vi "UI - BASLER - SINGLE MOTOR high accuracy.vi"() -> ()   [LabVIEW 2015]
uses:
  <vilib>/Utility/miscctls.llb/LVBoundsTypeDef.ctl
  Globals.vi
panel:
  in  "Correlate":bool
  in  "show":bool
  out "merged":picture
  out "fileNameFIBSEM":path
  out "fileNameMergedOPT":path
  in  "Colour 2":u16(ring)=1 items=["561 nm", "488 nm", "404 nm", ""]
  in  "Colour 1":u16(ring) items=["561 nm", "488 nm", "404 nm", ""]
  in  "Two lambda":bool
  in  "abort":bool
  in  "Two lambda old2":bool
  in  "ON/OFF":bool
  in  "Power %":dbl(slide) min=0.0 max=100.0 step=0.1 scale=0.0..100.0 scale format="%1_1f"
  in  "Colour":u16(ring) items=["561 nm", "488 nm", "404 nm", ""]
  in  "moveLAMELLA":bool
  in  "moveFIB":bool
  in  "moveOPT":bool
  in  "Save LAMELLA position":bool
  in  "Save FIB position":bool
  in  "Save OPT position":bool
  in  "Quit TCP":bool
  in  "Grab Image":bool
  out "done":string
  out "data out":string
  out "length":i32
  in  "Grab FIB-SEM":bool
  in  "error Obis":errorcluster
  out "Ready":bool
  in  "moveToOPT":bool
  in  "moveToFIB":bool
  in  "DY mm":dbl=-0.186 format="%.3f"
  in  "DX mm":dbl=49.919 format="%.3f"
  in  "yo":i32=1920
  in  "xo":i32=1200
  in  "yc":i32=2048
  in  "xc":i32=3072
  out "Intensity FIB-SEM":i32[][](graph) caption="Intensity Graph"
  in  "Path to Autoscript":path=path "C:/Program Files/Python35/envs/AutoScript/python.exe"
  in  "FIB/SEM":bool
  in  "Dwell time us":dbl=0.5 format="%#_6f"
  in  "Grab FIB-SEM OLD":bool
  out "wav 1":string
  out "Power":dbl
  in  "Power L1 %":i32(slide) scale=0.0..100.0
  out "LASmouseDOWN":bool
  out "Power1max":dbl
  out "Power1min":dbl
  out "PowerNom1":dbl
  out "lambda":dbl
  out "Obis out":refnum<visa-resource-name>
  in  "baud rate Obis":u32=9600
  out "Message Obis":string
  in  "ON/OFF 3":bool
  out "Obis":bool
  out "L1":bool
  in  "Laser":refnum<visa-resource-name>="COM11"
  out "commando":string
  out "fileName":path
  in  "File Prefix":string="embryo_561nm_"
  out "iii":i32
  in  "StepZ":dbl=1.0 format="%#.3g"
  in  "Nz":i32=50
  in  "startZ":i32=-8000 format="%.3f"
  in  "DIR Series":string="embryo_"
  in  "Scan":bool
  out "Intensity OPT":i32[][](graph) caption="Intensity Graph"
  out "pythonOut":string
  in  "Two lambda grab OLD":bool
  in  "Grab Image OLD":bool
  in  "Path to Python.exe":path=path "C:/Program Files/WinPython-64bit-3.5.4.0Qt5/python-3.5.4.amd64/python.exe"
  in  "Exposure ms":i32=500
  out "Right":bool
  out "Left":bool
  out "Path series":path
  out "date/time string":string="15:37"
  out "systemIndexOut":u32
  out "Path":path=path "C:/Users/Admin/MICROSCOPE/BASLER"
  in  "dz um":dbl=10.0 format="%.3f"
  out "status Z":T1(ring)
  in  "z um":dbl format="%.3f"
  in  "HOME":bool
  in  "STOP":bool
  out "moving":bool
  out "error stage":errorcluster
  out "Z Known?":bool
  in  "System Locator":string="usb:id:199871837"
  # "must be 3.5 for pypylon and basler"
  # "must be 3.5 for pypylon and basler"
  # "×"
  # "×"
  # "from FIB to OPT"
  # "from OPT to FIB"
  # "SEM"
  # "FIB"
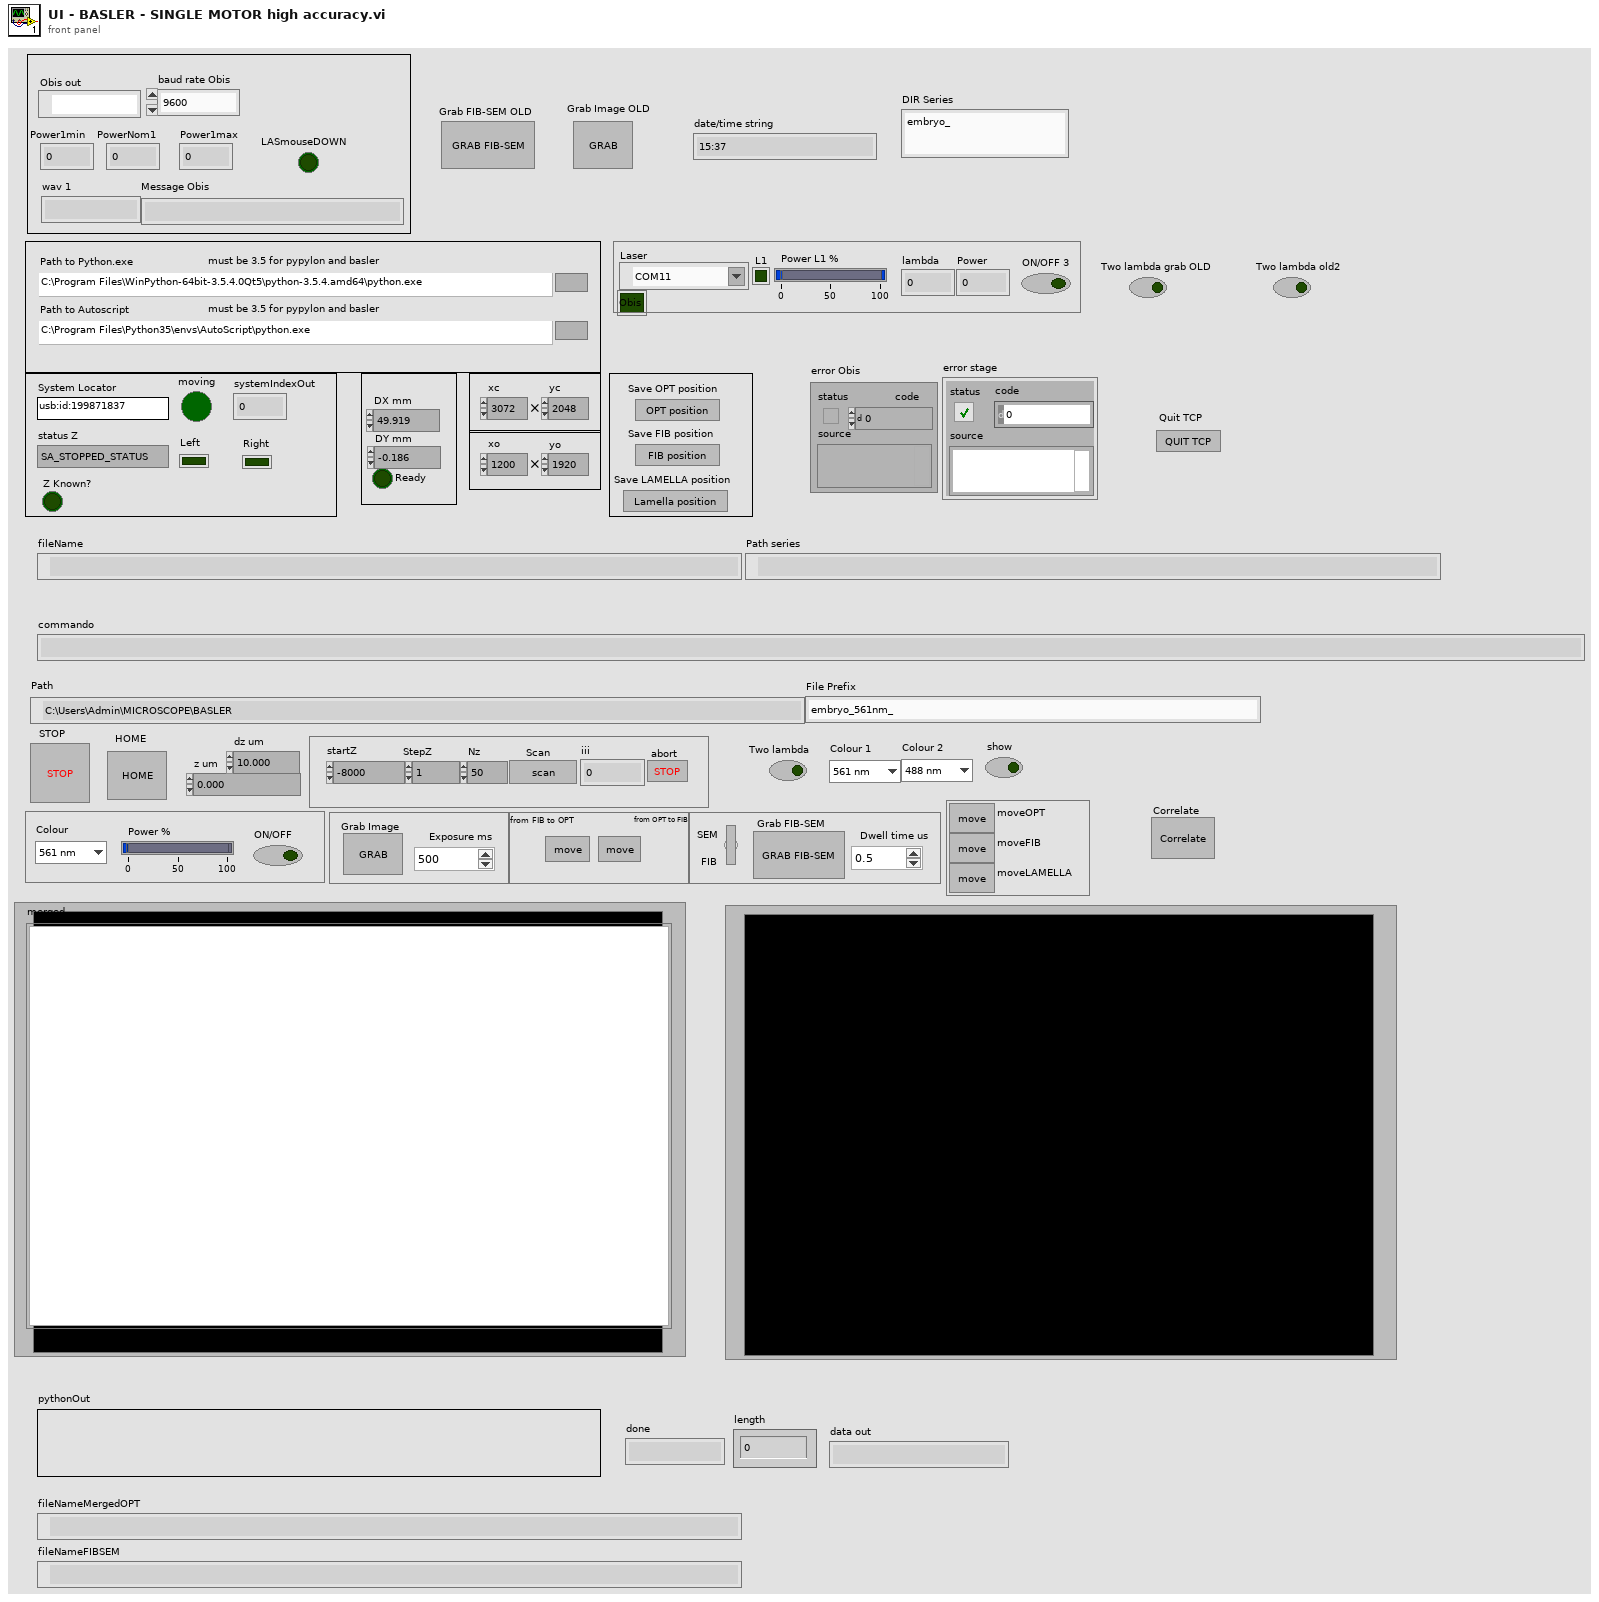
[diagram p1: front panel]
types:
  T1 = enum32{"SA_STOPPED_STATUS", "SA_STEPPING_STATUS", "SA_SCANNING_STATUS", "SA_HOLDING_STATUS", "SA_TARGET_STATUS", "SA_MOVE_DELAY_STATUS", "SA_CALIBRATING_STATUS", "SA_FINDING_REF_STATUS", "SA_OPENING_STATUS"}
  T2 = typedef "LVBoundsTypeDef.ctl" = cluster{"Width":u32, "Height":u32}
  T3 = enum32{"SA_FORWARD_DIRECTION", "SA_BACKWARD_DIRECTION", "SA_FORWARD_BACKWARD_DIRECTION", "SA_BACKWARD_FORWARD_DIRECTION"}
  T4 = typedef "eventvkey.ctl" = enum16{"ASCII", "Enter", "Return", "Shift", "Ctrl", "Alt", "Cmd", "Opt", "Caps", "NumLock", "Clear", "Break", "Up", "Down", "Left", "Right", "Insert", "Delete", "Home", "End", "PageUp", "PageDown", "Escape", "Help", "Pause", "ScrollLock", "F1", "F2", "F3", "F4", "F5", "F6", "F7", "F8", "F9", "F10", "F11", "F12", "F13", "F14", "F15", "F16", "F17", "F18", "F19", "F20", "F21", "F22", "F23", "F24", "Play", "VolumeUp", "VolumeDown", "Mute", "Two Byte Char"}
  T5 = typedef "imagedata.ctl" = cluster{"image type":i32, "image depth":i32, "image":u8[], "mask":u8[], "colors":u32[], "Rectangle":cluster{"left":i16, "top":i16, "right":i16, "bottom":i16}}
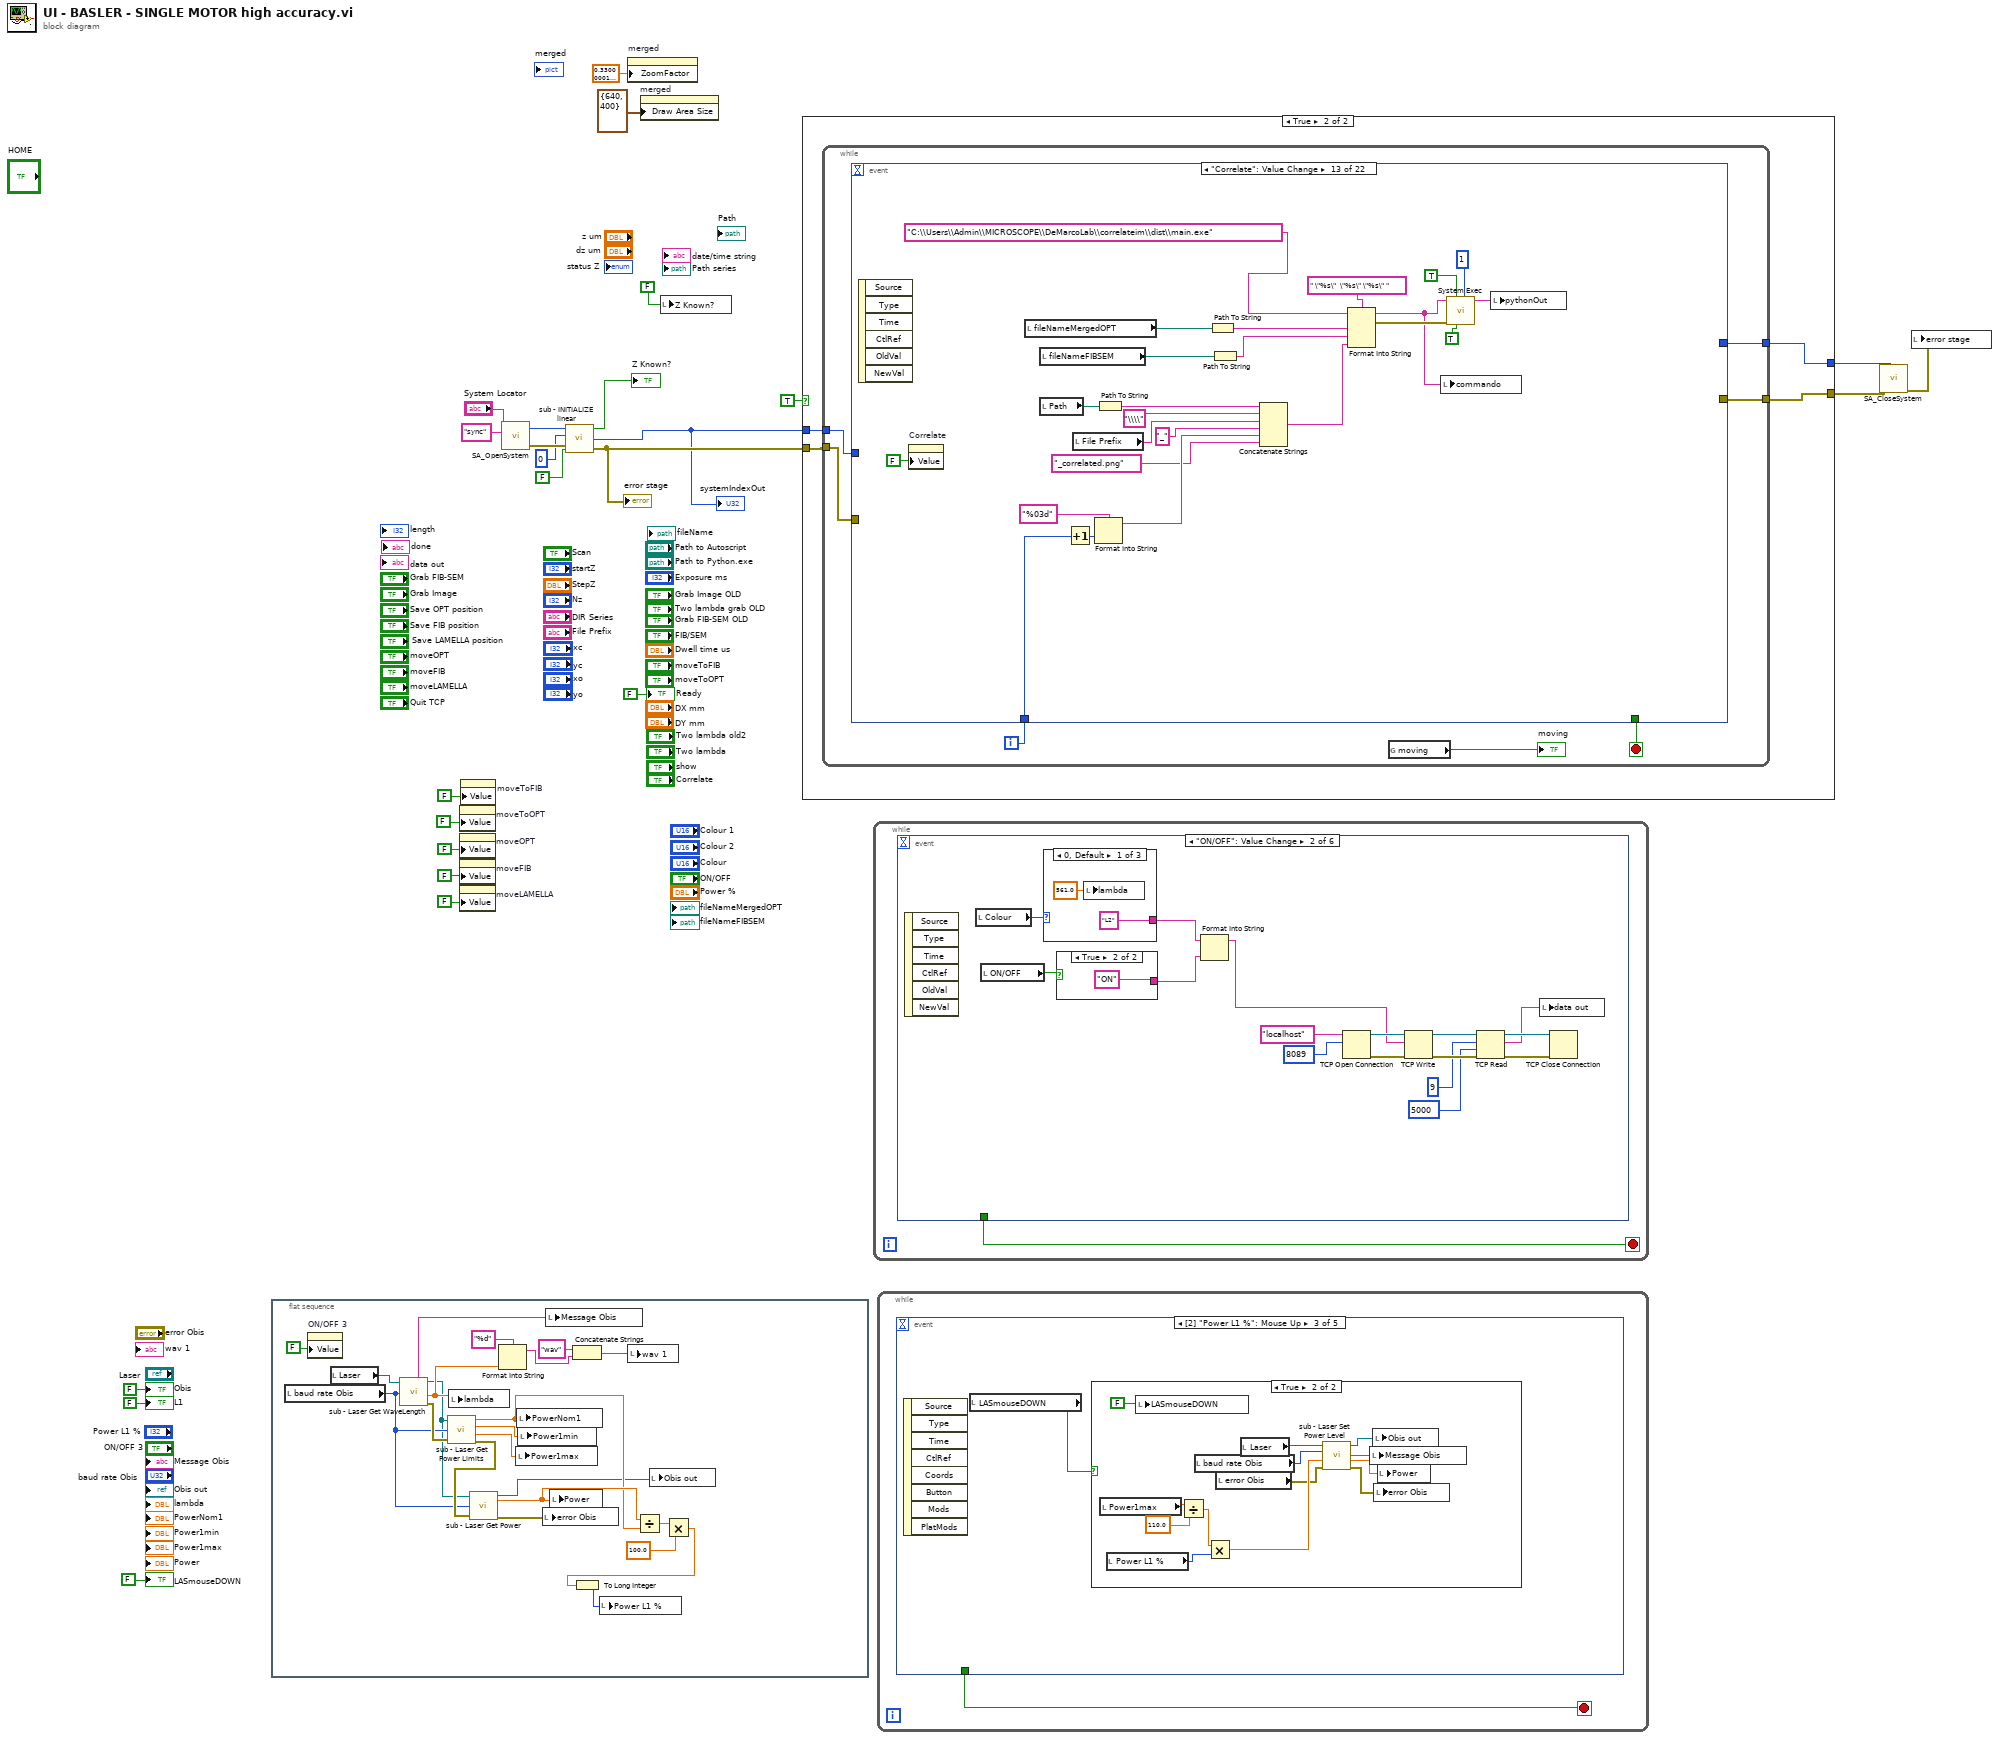
[diagram p0: block diagram]
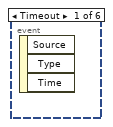
[diagram p2: hidden frame]
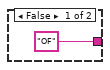
[diagram p3: hidden frame]
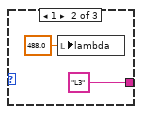
[diagram p4: hidden frame]
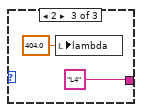
[diagram p5: hidden frame]
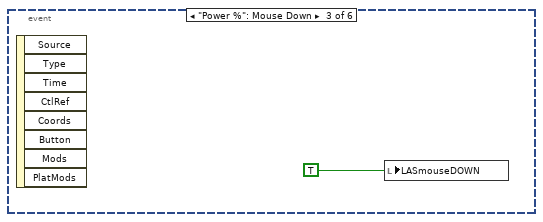
[diagram p6: hidden frame]
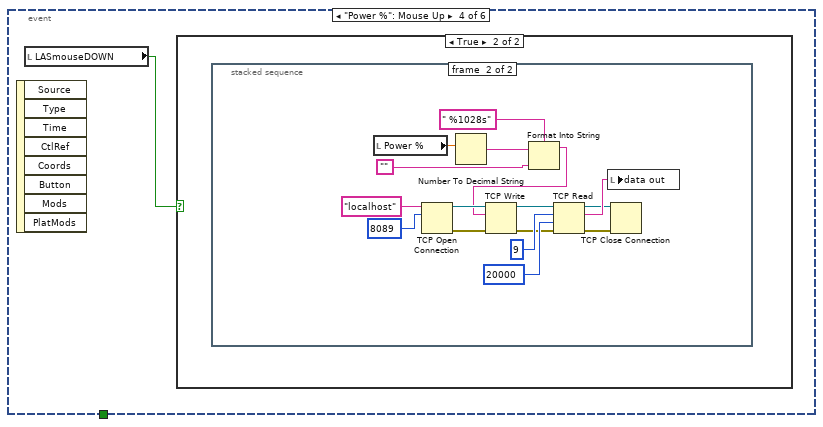
[diagram p7: hidden frame]
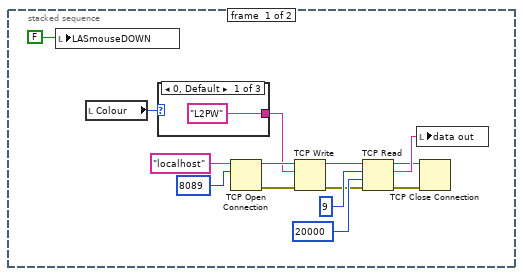
[diagram p9: hidden frame]
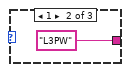
[diagram p10: hidden frame]
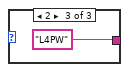
[diagram p11: hidden frame]
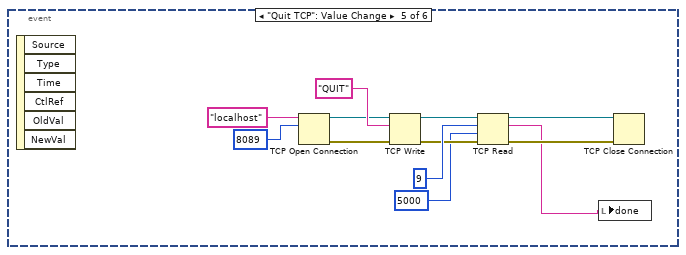
[diagram p12: hidden frame]
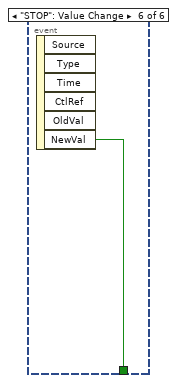
[diagram p13: hidden frame]
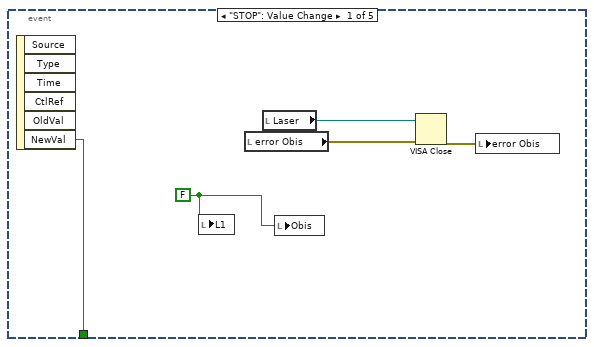
[diagram p14: hidden frame]
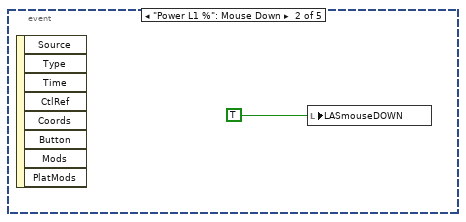
[diagram p15: hidden frame]
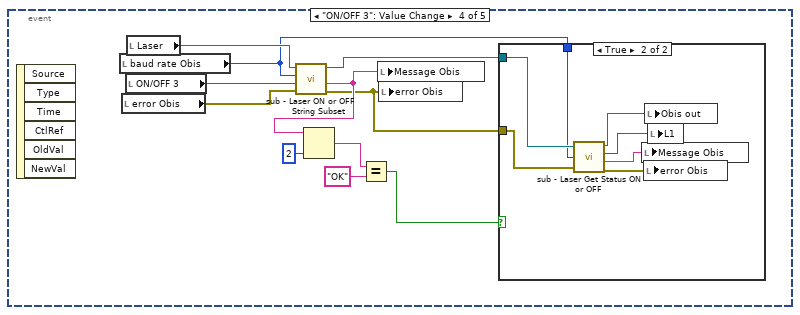
[diagram p17: hidden frame]
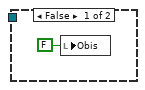
[diagram p18: hidden frame]
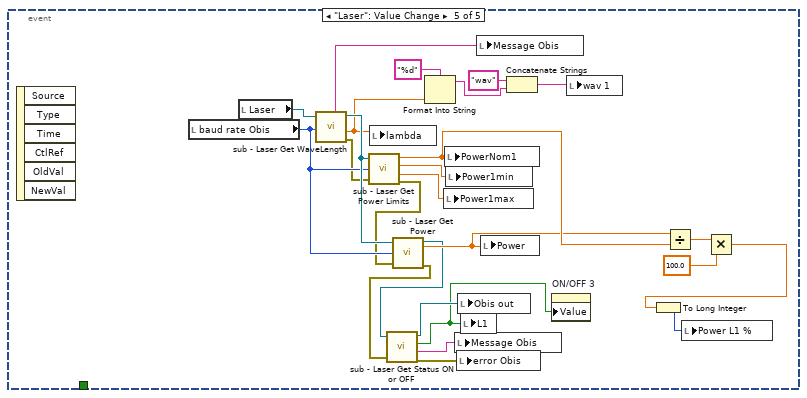
[diagram p19: hidden frame]
diagram:
  n1 = flat-sequence {
    frame #0 {
      n2 = local read "baud rate Obis"() -> (w39:u32)
      n3 = property on="ON/OFF 3" class="Bool (strict)"("Value"=FALSE ("L1 ON/OFF")) -> ()  [unwired: 2 in, 2 out]
      n4 = local read "Laser"() -> (w47:refnum<visa-resource-name>)
      n5 = call "sub - Laser Get WaveLength.vi"("VISA resource name"=w47, "baud rate (9600)"=w39) -> ("reference out"=w28:refnum<visa-resource-name>, "wavelength"=w31:dbl, "error out"=w44:errorcluster, "message"=w45:string)  [unwired: 1 in, 1 out]
      n6 = call "sub - Laser Get Power Limits.vi"("VISA resource name"=w28, "baud rate (9600)"=w39, "error in (no error)"=w44) -> ("powerNominal"=w37:dbl, "powerMin"=w43:dbl, "powerMax"=w42:dbl, "error out"=w41:errorcluster)  [unwired: 1 out]
      n7 = local write "lambda"(w31) -> ()
      n8 = call "sub - Laser Get Power.vi"("VISA resource name"=w28, "baud rate (9600)"=w39, "error in (no error)"=w41) -> ("reference out"=w26:refnum<visa-resource-name>, "Power"=w38:dbl, "error out"=w40:errorcluster)  [unwired: 2 out]
      n9 = Format Into String(format string="%d", w31) -> (resulting string=w27:string)  [unwired: 2 in, 1 out]
      n10 = local write "Power1max"(w42) -> ()
      n11 = local write "PowerNom1"(w37) -> ()
      n12 = local write "Power1min"(w43) -> ()
      n13 = local write "error Obis"(w40) -> ()
      n14 = local write "Message Obis"(w45) -> ()
      n15 = local write "Power"(w38) -> ()
      n16 = Concatenate Strings("wav" ("string"), w27) -> (w29:string)
      n17 = local write "wav 1"(w29) -> ()
      n18 = Divide(x=w38, y=w37) -> (x/y=w36:dbl)
      n19 = local write "Obis out"(w26) -> ()
      n20 = Multiply(x=w36, y=100.0) -> (x*y=w33:dbl)
      n21 = To Long Integer(number=w33) -> (32bit integer=w34:i32)
      n22 = local write "Power L1 %"(w34) -> ()
    }
  }
  n23 = property on="moveToOPT" class="Bool (strict)"("Value"=FALSE ("moveToOPT")) -> ()  [unwired: 2 in, 2 out]
  n24 = property on="moveOPT" class="Bool (strict)"("Value"=FALSE ("moveOPT")) -> ()  [unwired: 2 in, 2 out]
  n25 = property on="moveFIB" class="Bool (strict)"("Value"=FALSE ("moveFIB")) -> ()  [unwired: 2 in, 2 out]
  n26 = property on="moveLAMELLA" class="Bool (strict)"("Value"=FALSE ("moveLAMELLA")) -> ()  [unwired: 2 in, 2 out]
  n27 = property on="moveToFIB" class="Bool (strict)"("Value"=FALSE ("moveToFIB")) -> ()  [unwired: 2 in, 2 out]
  n28 = call <vilib>:"SA_OpenSystem.vi"("options"="sync", "systemLocator"="System Locator") -> ("error out"=w19:errorcluster, "systemIndexOut"=w20:u32)  [unwired: 8 in]
  n29 = call "sub - INITIALIZE linear.vi"("Zero?"=FALSE, "error in (no error)"=w19, "channelIndex"=u32 0, "systemIndex"=w20) -> ("error out"=w15:errorcluster, "systemIndexOut"=w14:u32, "Known?"=→"Z Known?":bool)
  "error stage" <- w15
  "systemIndexOut" <- w14
  n30 = property on="merged" class="Pict"("ZoomFactor"=sgl 0.33 ("Zoom Factor")) -> ()  [unwired: 2 in, 2 out]
  n31 = property on="merged" class="Pict"("Draw Area Size"=T2 {"Width"=640, "Height"=400}) -> ()  [unwired: 2 in, 2 out]
  n32 = local write "Z Known?"(FALSE ("X Known?")) -> ()
  n33 = case shown="True" TRUE {
    tunnel: w14 -> [w49 w53]
    tunnel: [w49 w51] -> w24
    tunnel: w15 -> [w48 w52]
    tunnel: [w48 w50] -> w23
    frame False {
    }
    frame True {
      n34 = while {
        tunnel: w53 -> [w59]
        tunnel: w52 -> [w56]
        tunnel: [w58] -> w51
        tunnel: [w57] -> w50
        i -> [w54]
        stop <- w60 stop-if-true
        n35 = event shown="[12] \"Correlate\": Value Change" {
          selector: _ -> [_ _ _ _ _ _ _ _ _ _ _ _ _ _ _ _ _ _ _ _ _ _]
          dyn-events: _ -> [_ _ _ _ _ _ _ _ _ _ _ _ _ _ _ _ _ _ _ _ _ _]
          timeout: _ -> [_ _ _ _ _ _ _ _ _ _ _ _ _ _ _ _ _ _ _ _ _ _]
          tunnel: [_ _ TRUE _ _ _ _ _ _ _ _ _ _ _ _ _ _ _ _ _ _ FALSE] -> w60
          tunnel: w59 -> [w62 w95 w117 _ _ _ _ _ _ _ _ _ _ _ _ _ _ _ _ _ _ w1778]
          tunnel: w56 -> [w61 w98 w118 _ _ _ _ _ _ _ _ _ _ _ _ _ _ _ _ _ _ w1779]
          tunnel: [_ _ w115 _ _ _ _ _ _ _ _ _ _ _ _ _ _ _ _ _ _ w1778] -> w58
          tunnel: [_ _ w113 _ _ _ _ _ _ _ _ _ _ _ _ _ _ _ _ _ _ _] -> w57
          tunnel: w54 -> [_ _ _ _ _ _ w415 w577 _ w1112 w1440 _ w1577 _ _ _ _ _ _ _ _ _]
          event Key Down {
            n36 = event-data() -> ("VKey"=w63:T4)  [unwired: 1 in, 9 out]
            n37 = case shown="\"Left\"" w63 {
              tunnel: w62 -> [w65 w68 w83]
              tunnel: w61 -> [w64 w66 w81]
              tunnel: [w65 w75 w89] -> _
              tunnel: [w64 w74 w88] -> _
              frame "ASCII", Default {
              }
              frame "Right" {
                n38 = local read "dz um"() -> (w73:dbl)
                n39 = Multiply(x=w73, y=-1) -> (x*y=w67:dbl)
                n40 = call "sub - GoTo Position RELATIVE - HIGH ACCURACY.vi"("error in"=w66, "dx um"=w67, "channelIndex"=u32 0, "systemIndex"=w68) -> ("error out"=w72:errorcluster, "position out um"=w69:dbl, "status"=w71:T1)  [unwired: 2 out]
                n41 = local write "status Z"(w71) -> ()
                n42 = property on="z um" class="DigNum (strict)"("Value"=w69) -> ()  [unwired: 2 in, 2 out]
                n43 = global write "Globals.vi" "X"(w69) -> ()
                n44 = flat-sequence {
                  tunnel: w68 -> [w80]
                  tunnel: [w80] -> w75
                  tunnel: w72 -> [w79]
                  tunnel: [w79] -> w74
                  frame #0 {
                    n45 = local write "Left"(FALSE) -> ()
                  }
                }
                "Left" <- TRUE ("Boolean 2")
              }
              frame "Left" {
                n46 = local read "dz um"() -> (w82:dbl)
                n47 = call "sub - GoTo Position RELATIVE - HIGH ACCURACY.vi"("error in"=w81, "dx um"=w82, "channelIndex"=u32 0, "systemIndex"=w83) -> ("error out"=w86:errorcluster, "position out um"=w84:dbl, "status"=w87:T1)  [unwired: 2 out]
                n48 = local write "status Z"(w87) -> ()
                n49 = global write "Globals.vi" "X"(w84) -> ()
                n50 = property on="z um" class="DigNum (strict)"("Value"=w84) -> ()  [unwired: 2 in, 2 out]
                n51 = flat-sequence {
                  tunnel: w83 -> [w92]
                  tunnel: [w92] -> w89
                  tunnel: w86 -> [w91]
                  tunnel: [w91] -> w88
                  frame #0 {
                    n52 = local write "Right"(FALSE) -> ()
                  }
                }
                "Right" <- TRUE ("Boolean 2")
              }
            }
          }
          event "z um": Value Change {
            n53 = event-data() -> ()  [unwired: 1 in, 6 out]
            n54 = local read "z um"() -> (w97:dbl)
            n55 = call "sub - GoTo Position Absolute ABSOLUTE - HIGH ACCURACY.vi"("error in"=w98, "Position End um"=w97, "channelIndex"=u32 0, "systemIndex"=w95) -> ("error out"=w99:errorcluster, "position out um"=w94:dbl, "status"=w100:T1)  [unwired: 2 out]
            n56 = local write "error stage"(w99) -> ()
            n57 = local write "status Z"(w100) -> ()
            n58 = property on="z um" class="DigNum (strict)"("Value"=w94) -> ()  [unwired: 2 in, 2 out]
          }
          event "STOP": Value Change {
            n59 = event-data() -> ()  [unwired: 1 in, 6 out]
            n60 = flat-sequence {
              tunnel: w118 -> [w125]
              tunnel: w117 -> [w124]
              tunnel: [w122] -> w116
              tunnel: [w121] -> w114
              tunnel: [w140] -> w115
              tunnel: w116 -> [w140]
              tunnel: [w139] -> w113
              tunnel: w114 -> [w139]
              frame #0 {
                w123 = u32 0 ("channelIndex")
                n61 = call <vilib>:"SA_FindReferenceMark_S.vi"("channelIndex"=w123, "systemIndex"=u32 777, "error in (no error)"=w125, "autoZero"=enum32{"SA_NO_AUTO_ZERO", "SA_AUTO_ZERO"}."SA_AUTO_ZERO", "holdTime"=u32 0, "direction"=T3."SA_FORWARD_DIRECTION") -> ("error out"=w129:errorcluster)  [unwired: 5 in]
                n62 = while {
                  tunnel: w124 -> [w135]
                  tunnel: w123 -> [w137]
                  shift-right: [w136] -> w121
                  shift-left: w129 -> [w138]
                  tunnel: [w135] -> w122
                  stop <- w131 stop-if-true
                  n63 = call <vilib>:"SA_GetStatus_S.vi"("channelIndex"=w137, "systemIndex"=u32 777, "error in (no error)"=w138) -> ("error out"=w136:errorcluster, "status"=w134:T1)  [unwired: 7 in]
                  n64 = Equal?(x=T1."SA_STOPPED_STATUS" ("y"), y=w134) -> (x = y?=w131:bool)
                  n65 = Wait (ms)(milliseconds to wait=u32 100) -> ()  [unwired: 1 out]
                }
              }
              frame #1 {
                n66 = global write "Globals.vi" "Stop"("STOP") -> ()
              }
            }
            n67 = TCP Open Connection(address="localhost", remote port or service name=u16 8089) -> (connection ID=w105:refnum<k5>, error out=w104:errorcluster)  [unwired: 3 in]
            n68 = TCP Write(connection ID=w105, data in="QUIT", error in (no error)=w104) -> (connection ID out=w110:refnum<k5>, error out=w109:errorcluster)  [unwired: 1 in, 1 out]
            n69 = TCP Read(connection ID=w110, bytes to read=9, error in (no error)=w109, 9:5000 ("timeout ms (25000)")) -> (connection ID out=w103:refnum<k5>, data out=w101:string, error out=w102:errorcluster)  [unwired: 1 in]
            n70 = local write "done"(w101) -> ()
            n71 = TCP Close Connection(connection ID=w103, error in (no error)=w102) -> ()  [unwired: 1 in, 2 out]
          }
          event "Grab Image OLD": Value Change {
            # "3"
            n72 = event-data() -> ()  [unwired: 1 in, 6 out]
            n73 = local read "Path to Autoscript"() -> (w157:path)
            n74 = local read "Exposure ms"() -> (w155:i32)
            n75 = Multiply(x=w155, y=1000.0) -> (x*y=w154:dbl)
            n76 = Path To String(path=w157) -> (string=w161:string)
            n77 = To Long Integer(number=w154) -> (32bit integer=w153:i32)
            n78 = Format Into String(format string=" \"%s\" %d", initial string=w161, "C:\\Users\\Admin\\MICROSCOPE\\PyPylon_3.5\\camera.py" ("Path to Function"), w153) -> (resulting string=w142:string, error out=w160:errorcluster)  [unwired: 1 in]
            n79 = flat-sequence {
              tunnel: w152 -> [w165]
              tunnel: [w167] -> w146
              frame #0 {
                n80 = Wait (ms)(milliseconds to wait=u32 10) -> ()  [unwired: 1 out]
                "pythonOut" <- w165
              }
              frame #1 {
                n81 = property on="Grab Image OLD" class="Bool (strict)"("Value"=FALSE ("Grab Image")) -> ()  [unwired: 2 in, 2 out]
                n82 = Read from Text File(file (use dialog)=path "C:/Users/Admin/MICROSCOPE/BASLER/dataout.txt" ("file path (dialog if empty)")) -> (text=w167:string)  [unwired: 3 in, 3 out]
              }
            }
            n83 = local write "commando"(w142) -> ()
            n84 = call <vilib>:"System Exec.vi"("run minimized? (F)"=TRUE, "wait until completion? (T)"=TRUE, "error in (no error)"=w160, "command line"=w142) -> ("standard output"=w152:string)  [unwired: 4 in, 3 out]
            n85 = Spreadsheet String To Array(delimiter (Tab)=" ", format string="", spreadsheet string=w146) -> (array=w150:dbl[][])  [unwired: 1 in]
            n86 = local read "yo"() -> (w144:i32)
            n87 = local read "xo"() -> (w143:i32)
            n88 = To Long Integer(number=w150) -> (32bit integer=w149:i32[][])
            n89 = Reshape Array(w149, w144, w143) -> (w151:i32[][])
            n90 = To Long Integer(number=w151) -> (32bit integer=→"Intensity OPT":i32[][])
          }
          event "Scan": Value Change {
            n91 = event-data() -> ()  [unwired: 1 in, 6 out]
            n92 = property on="Scan" class="Bool (strict)"("Value"=FALSE ("Scan")) -> ()  [unwired: 2 in, 2 out]
            n93 = stacked-sequence {
              frame #0 {
                n94 = local read "lambda"() -> (w173:dbl)
                n95 = local read "File Prefix"() -> (w175:string)
                n96 = local read "Path"() -> (w186:path)
                n97 = Number To Decimal String(number=w173) -> (decimal integer string=w172:string)  [unwired: 1 in]
                n98 = Path To String(path=w186) -> (string=w189:string)
                n99 = local read "systemIndexOut"() -> (w178:u32)
                n100 = Format Date/Time String(time format string (%c)="%Y_%m_%d_%H_%M_%S") -> (date/time string=w170:string)  [unwired: 2 in]
                n101 = local read "error stage"() -> (w177:errorcluster)
                n102 = Concatenate Strings(w189, "\\\\" ("format string"), w175, "_SERIES_" ("format string"), w172, "nm__" ("format string"), w170) -> (w188:string)
                n103 = local write "date/time string"(w170) -> ()
                n104 = String To Path(string=w188) -> (path=w187:path)
                n105 = call <vilib>:"Check if File or Folder Exists.vi"("path"=w187) -> ("file or folder exists?"=w185:bool, "dup path"=w184:path)  [unwired: 8 in, 1 out]
                n106 = case shown="False" w185 {
                  tunnel: w184 -> [w192 w194]
                  tunnel: [w193 w194] -> w191
                  frame False {
                    n107 = Create Folder(path (use dialog)=w192) -> (created path=w193:path)  [unwired: 2 in, 2 out]
                  }
                  frame True {
                  }
                }
                n108 = call <vilib>:"SA_GetPosition_S.vi"("channelIndex"=u32 0, "systemIndex"=w178, "error in (no error)"=w177) -> ("error out"=w176:errorcluster, "position"=w181:i32)  [unwired: 7 in]
                n109 = Divide(x=w181, y=1000) -> (x/y=w182:dbl)
                n110 = local write "error stage"(w176) -> ()
                n111 = local write "startZ"(w182) -> ()
                n112 = local write "Path series"(w191) -> ()
              }
              frame #1 {
                n113 = local read "Nz"() -> (w195:i32)
                n114 = for {
                  N: w195 -> [_]
                  i -> [w197]
                  stop <- "abort" stop-if-true
                  n115 = stacked-sequence {
                    frame #0 {
                      # "Move to the position"
                      n116 = local read "StepZ"() -> (w206:dbl)
                      n117 = local read "systemIndexOut"() -> (w200:u32)
                      n118 = local read "error stage"() -> (w203:errorcluster)
                      n119 = local read "iii"() -> (w205:i32)
                      n120 = local read "startZ"() -> (w204:i32)
                      n121 = Multiply(x=w205, y=w206) -> (x*y=w207:dbl)
                      n122 = Add(x=w204, y=w207) -> (x+y=w199:dbl)
                      n123 = call "sub - GoTo Position Absolute ABSOLUTE - HIGH ACCURACY.vi"("error in"=w203, "Position End um"=w199, "channelIndex"=u32 0, "systemIndex"=w200) -> ("position out um"=w198:dbl, "status"=w201:T1)  [unwired: 3 out]
                      n124 = local write "status Z"(w201) -> ()
                      n125 = global write "Globals.vi" "X"(w198) -> ()
                      n126 = property on="z um" class="DigNum (strict)"("Value"=w198) -> ()  [unwired: 2 in, 2 out]
                    }
                    frame #1 {
                      n127 = local read "Path series"() -> (w220:path)
                      n128 = property on="z um" class="DigNum (strict)"() -> ("Value"=w215:dbl)  [unwired: 2 in, 2 out]
                      n129 = local read "iii"() -> (w218:i32)
                      n130 = Increment(x=w218) -> (x+1=w219:i32)
                      n131 = Path To String(path=w220) -> (string=w208:string)
                      n132 = String To Path(string=w208) -> (path=w226:path)
                      n133 = Format Into String(format string="%06f", w215) -> (resulting string=w231:string)  [unwired: 2 in, 1 out]
                      n134 = Format Into String(format string="%03d", w219) -> (resulting string=w217:string)  [unwired: 2 in, 1 out]
                      n135 = call <vilib>:"Check if File or Folder Exists.vi"("path"=w226) -> ("file or folder exists?"=w225:bool, "dup path"=w224:path)  [unwired: 8 in, 1 out]
                      n136 = case shown="False" w225 {
                        tunnel: w224 -> [w232 w234]
                        tunnel: [w233 w234] -> w221
                        frame False {
                          n137 = Create Folder(path (use dialog)=w232) -> (created path=w233:path)  [unwired: 2 in, 2 out]
                        }
                        frame True {
                        }
                      }
                      n138 = Concatenate Strings("_" ("string"), "_" ("string"), w217, "_" ("string"), w231) -> (w211:string)
                      n139 = local read "File Prefix"() -> (w213:string)
                      n140 = Path To String(path=w221) -> (string=w223:string)
                      n141 = Concatenate Strings(w223, "\\\\" ("format string"), w213, "__" ("format string"), w211, ".bmp" ("format string")) -> (w222:string)
                      n142 = String To Path(string=w222) -> (path=w209:path)
                      n143 = local write "fileName"(w209) -> ()
                    }
                    frame #2 {
                      n144 = case shown="True" FALSE {
                        frame False {
                        }
                        frame True {
                          # "U S E   TCP    to send commands"
                          # "OLD WAY TO ACQUIRE IMAGE"
                          n145 = local read "Path series"() -> (w250:path)
                          n146 = local read "Path to Python.exe"() -> (w240:path)
                          n147 = local read "fileName"() -> (w251:path)
                          n148 = local read "Exposure ms"() -> (w238:i32)
                          n149 = Path To String(path=w250) -> (string=w252:string)
                          n150 = Path To String(path=w251) -> (string=w253:string)
                          n151 = Multiply(x=w238, y=1000.0) -> (x*y=w237:dbl)
                          n152 = Path To String(path=w240) -> (string=w245:string)
                          n153 = To Long Integer(number=w237) -> (32bit integer=w236:i32)
                          n154 = Format Into String(format string=" \"%s\" %d \"%s\" \"%s\" \"%s\"", initial string=w245, "C:\\Users\\Admin\\MICROSCOPE\\PyPylon_3.5\\camera.py" ("Path to Function"), w236, "save" ("format string"), w252, w253) -> (resulting string=w242:string, error out=w244:errorcluster)  [unwired: 1 in]
                          "commando" <- w242
                          n155 = call <vilib>:"System Exec.vi"("run minimized? (F)"=TRUE, "wait until completion? (T)"=TRUE, "error in (no error)"=w244, "command line"=w242) -> ("standard output"=w248:string)  [unwired: 4 in, 3 out]
                          n156 = local write "pythonOut"(w248) -> ()
                        }
                      }
                    }
                    frame #3 {
                      n157 = TCP Open Connection(address="localhost", remote port or service name=u16 8089) -> (connection ID=w260:refnum<k5>, error out=w259:errorcluster)  [unwired: 3 in]
                      n158 = TCP Write(connection ID=w260, data in="_OPT" ("format string"), error in (no error)=w259) -> (connection ID out=w265:refnum<k5>, error out=w264:errorcluster)  [unwired: 1 in, 1 out]
                      n159 = TCP Read(connection ID=w265, bytes to read=9, error in (no error)=w264, 9:20000 ("timeout ms (25000)")) -> (connection ID out=w258:refnum<k5>, data out=w255:string, error out=w257:errorcluster)  [unwired: 1 in]
                      n160 = TCP Close Connection(connection ID=w258, error in (no error)=w257) -> ()  [unwired: 1 in, 2 out]
                      n161 = local write "data out"(w255) -> ()
                    }
                    frame #4 {
                      n162 = flat-sequence {
                        frame #0 {
                          n163 = TCP Open Connection(address="localhost", remote port or service name=u16 8089) -> (connection ID=w271:refnum<k5>, error out=w270:errorcluster)  [unwired: 3 in]
                          n164 = TCP Write(connection ID=w271, data in="EXPS", error in (no error)=w270) -> (connection ID out=w276:refnum<k5>, error out=w275:errorcluster)  [unwired: 1 in, 1 out]
                          n165 = TCP Read(connection ID=w276, bytes to read=9, error in (no error)=w275, 9:20000 ("timeout ms (25000)")) -> (connection ID out=w269:refnum<k5>, data out=w266:string, error out=w268:errorcluster)  [unwired: 1 in]
                          n166 = local write "data out"(w266) -> ()
                          n167 = TCP Close Connection(connection ID=w269, error in (no error)=w268) -> ()  [unwired: 1 in, 2 out]
                        }
                        frame #1 {
                          n168 = local read "Exposure ms"() -> (w280:i32)
                          n169 = TCP Open Connection(address="localhost", remote port or service name=u16 8089) -> (connection ID=w287:refnum<k5>, error out=w288:errorcluster)  [unwired: 3 in]
                          n170 = Number To Decimal String(number=w280) -> (decimal integer string=w279:string)  [unwired: 1 in]
                          n171 = Format Into String(format string=" %4s", initial string=w279, "") -> (resulting string=w281:string)  [unwired: 1 in, 1 out]
                          n172 = TCP Write(connection ID=w287, data in=w281, error in (no error)=w288) -> (connection ID out=w282:refnum<k5>, error out=w283:errorcluster)  [unwired: 1 in, 1 out]
                          n173 = TCP Read(connection ID=w282, bytes to read=9, error in (no error)=w283, 9:20000 ("timeout ms (25000)")) -> (connection ID out=w289:refnum<k5>, data out=w292:string, error out=w290:errorcluster)  [unwired: 1 in]
                          n174 = local write "data out"(w292) -> ()
                          n175 = TCP Close Connection(connection ID=w289, error in (no error)=w290) -> ()  [unwired: 1 in, 2 out]
                        }
                      }
                    }
                    frame #5 {
                      n176 = flat-sequence {
                        frame #0 {
                          n177 = TCP Open Connection(address="localhost", remote port or service name=u16 8089) -> (connection ID=w299:refnum<k5>, error out=w298:errorcluster)  [unwired: 3 in]
                          n178 = TCP Write(connection ID=w299, data in="_DIR", error in (no error)=w298) -> (connection ID out=w304:refnum<k5>, error out=w303:errorcluster)  [unwired: 1 in, 1 out]
                          n179 = TCP Read(connection ID=w304, bytes to read=9, error in (no error)=w303, 9:20000 ("timeout ms (25000)")) -> (connection ID out=w297:refnum<k5>, data out=w294:string, error out=w296:errorcluster)  [unwired: 1 in]
                          n180 = local write "data out"(w294) -> ()
                          n181 = TCP Close Connection(connection ID=w297, error in (no error)=w296) -> ()  [unwired: 1 in, 2 out]
                        }
                        frame #1 {
                          n182 = local read "fileName"() -> (w310:path)
                          n183 = Path To String(path=w310) -> (string=w308:string)
                          n184 = TCP Open Connection(address="localhost", remote port or service name=u16 8089) -> (connection ID=w316:refnum<k5>, error out=w317:errorcluster)  [unwired: 3 in]
                          n185 = Format Into String(format string=" %1028s", initial string=w308, "") -> (resulting string=w309:string)  [unwired: 1 in, 1 out]
                          n186 = TCP Write(connection ID=w316, data in=w309, error in (no error)=w317) -> (connection ID out=w311:refnum<k5>, error out=w312:errorcluster)  [unwired: 1 in, 1 out]
                          n187 = TCP Read(connection ID=w311, bytes to read=9, error in (no error)=w312, 9:20000 ("timeout ms (25000)")) -> (connection ID out=w318:refnum<k5>, data out=w321:string, error out=w319:errorcluster)  [unwired: 1 in]
                          n188 = local write "data out"(w321) -> ()
                          n189 = TCP Close Connection(connection ID=w318, error in (no error)=w319) -> ()  [unwired: 1 in, 2 out]
                        }
                      }
                    }
                    frame #6 {
                      n190 = TCP Open Connection(address="localhost", remote port or service name=u16 8089) -> (connection ID=w327:refnum<k5>, error out=w326:errorcluster)  [unwired: 3 in]
                      n191 = TCP Write(connection ID=w327, data in="IMGO", error in (no error)=w326) -> (connection ID out=w332:refnum<k5>, error out=w331:errorcluster)  [unwired: 1 in, 1 out]
                      n192 = TCP Read(connection ID=w332, bytes to read=9, error in (no error)=w331, 9:20000 ("timeout ms (25000)")) -> (connection ID out=w325:refnum<k5>, data out=w322:string, error out=w324:errorcluster)  [unwired: 1 in]
                      n193 = TCP Close Connection(connection ID=w325, error in (no error)=w324) -> ()  [unwired: 1 in, 2 out]
                      n194 = local write "data out"(w322) -> ()
                    }
                    frame #7 {
                      n195 = TCP Open Connection(address="localhost", remote port or service name=u16 8089) -> (connection ID=w340:refnum<k5>, error out=w339:errorcluster)  [unwired: 3 in]
                      n196 = TCP Write(connection ID=w340, data in="GETL", error in (no error)=w339) -> (connection ID out=w345:refnum<k5>, error out=w344:errorcluster)  [unwired: 1 in, 1 out]
                      n197 = TCP Read(connection ID=w345, bytes to read=20, error in (no error)=w344, 9:5000 ("timeout ms (25000)")) -> (connection ID out=w338:refnum<k5>, data out=w335:string, error out=w337:errorcluster)  [unwired: 1 in]
                      n198 = Decimal String To Number(string=w335) -> (number=w334:i32)  [unwired: 2 in, 1 out]
                      n199 = local write "data out"(w335) -> ()
                      n200 = TCP Close Connection(connection ID=w338, error in (no error)=w337) -> ()  [unwired: 1 in, 2 out]
                      n201 = local write "length"(w334) -> ()
                    }
                    frame #8 {
                      n202 = local read "length"() -> (w363:i32)
                      n203 = TCP Open Connection(address="localhost", remote port or service name=u16 8089) -> (connection ID=w361:refnum<k5>, error out=w362:errorcluster)  [unwired: 3 in]
                      n204 = TCP Write(connection ID=w361, data in="DATA", error in (no error)=w362) -> (connection ID out=w356:refnum<k5>, error out=w357:errorcluster)  [unwired: 1 in, 1 out]
                      n205 = TCP Read(connection ID=w356, bytes to read=w363, error in (no error)=w357, 9:5000 ("timeout ms (25000)")) -> (data out=w347:string)  [unwired: 1 in, 2 out]
                      n206 = Spreadsheet String To Array(delimiter (Tab)=" ", format string="", spreadsheet string=w347) -> (array=w353:dbl[][])  [unwired: 1 in]
                      n207 = local read "yo"() -> (w348:i32)
                      n208 = local read "xo"() -> (w349:i32)
                      n209 = To Long Integer(number=w353) -> (32bit integer=w352:i32[][])
                      n210 = Reshape Array(w352, w348, w349) -> (w354:i32[][])
                      n211 = To Long Integer(number=w354) -> (32bit integer=w364:i32[][])
                      n212 = local write "Intensity OPT"(w364) -> ()
                    }
                  }
                  "iii" <- w197
                }
              }
            }
          }
          event "Grab FIB-SEM OLD": Value Change {
            n213 = event-data() -> ()  [unwired: 1 in, 6 out]
            n214 = stacked-sequence {
              frame #0 {
                n215 = local read "FIB/SEM"() -> (w366:bool)
                n216 = case shown="True" w366 {
                  tunnel: ["_FIB_" ("format string") "_SEM_" ("format string")] -> w365
                  frame False {
                  }
                  frame True {
                  }
                }
                n217 = local read "File Prefix"() -> (w368:string)
                n218 = local read "Path"() -> (w372:path)
                n219 = Path To String(path=w372) -> (string=w375:string)
                n220 = Format Date/Time String(time format string (%c)="%Y_%m_%d_%H_%M_%S") -> (date/time string=w367:string)  [unwired: 2 in]
                n221 = Concatenate Strings(w375, "\\\\" ("format string"), w368, w365, w367) -> (w374:string)
                n222 = local write "date/time string"(w367) -> ()
                n223 = String To Path(string=w374) -> (path=w373:path)
                n224 = call <vilib>:"Check if File or Folder Exists.vi"("path"=w373) -> ("file or folder exists?"=w371:bool, "dup path"=w370:path)  [unwired: 8 in, 1 out]
                n225 = case shown="False" w371 {
                  tunnel: w370 -> [w380 w382]
                  tunnel: [w381 w382] -> w377
                  frame False {
                    n226 = Create Folder(path (use dialog)=w380) -> (created path=w381:path)  [unwired: 2 in, 2 out]
                  }
                  frame True {
                  }
                }
                n227 = local write "Path series"(w377) -> ()
              }
              frame #1 {
                n228 = local read "FIB/SEM"() -> (w389:bool)
                n229 = case shown="False" w389 {
                  tunnel: ["C:\\Users\\Admin\\MICROSCOPE\\pfib__GetFIBimage.py" ("Path to Function") "C:\\Users\\Admin\\MICROSCOPE\\pfib__GetSEMimage.py" ("Path to Function")] -> w388
                  frame False {
                  }
                  frame True {
                  }
                }
                n230 = local read "File Prefix"() -> (w387:string)
                n231 = local read "Path series"() -> (w397:path)
                n232 = local read "Path to Autoscript"() -> (w390:path)
                n233 = local read "Dwell time us"() -> (w384:dbl)
                n234 = Path To String(path=w397) -> (string=w398:string)
                n235 = Path To String(path=w390) -> (string=w394:string)
                n236 = Format Into String(format string=" \"%s\" %f \"%s\" \"%s\" \"%s\"", initial string=w394, w388, w384, w387, w398, "plot" ("Path to Function")) -> (resulting string=w385:string, error out=w393:errorcluster)  [unwired: 1 in]
                n237 = local write "commando"(w385) -> ()
                n238 = call <vilib>:"System Exec.vi"("expected output size  (4096)"=u32 1, "run minimized? (F)"=TRUE, "wait until completion? (T)"=TRUE, "error in (no error)"=w393, "command line"=w385) -> ("standard output"=w396:string)  [unwired: 3 in, 3 out]
                n239 = local write "pythonOut"(w396) -> ()
              }
              frame #2 {
                n240 = local read "FIB/SEM"() -> (w412:bool)
                n241 = property on="Grab FIB-SEM OLD" class="Bool (strict)"("Value"=FALSE ("Grab Image")) -> ()  [unwired: 2 in, 2 out]
                n242 = case shown="True" w412 {
                  tunnel: [path "C:/Users/Admin/MICROSCOPE/BASLER/dataoutFIB.txt" ("file path (dialog if empty)") path "C:/Users/Admin/MICROSCOPE/BASLER/dataoutSEM.txt" ("file path (dialog if empty)")] -> w411
                  frame False {
                  }
                  frame True {
                  }
                }
                n243 = local read "xc"() -> (w401:i32)
                n244 = local read "yc"() -> (w402:i32)
                n245 = Read from Text File(file (use dialog)=w411) -> (text=w403:string)  [unwired: 3 in, 3 out]
                n246 = Spreadsheet String To Array(delimiter (Tab)=" ", format string="", spreadsheet string=w403) -> (array=w408:dbl[][])  [unwired: 1 in]
                n247 = To Long Integer(number=w408) -> (32bit integer=w407:i32[][])
                n248 = Reshape Array(w407, w401, w402) -> (w409:i32[][])
                n249 = To Long Integer(number=w409) -> (32bit integer=→"Intensity FIB-SEM":i32[][])
              }
            }
          }
          event "Grab FIB-SEM": Value Change {
            n250 = event-data() -> ()  [unwired: 1 in, 6 out]
            n251 = stacked-sequence {
              tunnel: w415 -> [w419 _ _ _ _ _ _ _ _]
              frame #0 {
                n252 = local read "FIB/SEM"() -> (w424:bool)
                n253 = local read "Path"() -> (w428:path)
                n254 = case shown="True" w424 {
                  tunnel: ["_FIB_" ("format string") "_SEM_" ("format string")] -> w416
                  frame False {
                  }
                  frame True {
                  }
                }
                n255 = local read "File Prefix"() -> (w426:string)
                n256 = Path To String(path=w428) -> (string=w431:string)
                n257 = Increment(x=w419) -> (x+1=w420:i32)
                n258 = Format Into String(format string="%03d", w420) -> (resulting string=w417:string)  [unwired: 2 in, 1 out]
                n259 = Format Date/Time String(time format string (%c)="%Y_%m_%d_%H_%M_%S") -> (date/time string=w425:string)  [unwired: 2 in]
                n260 = local write "date/time string"(w425) -> ()
                n261 = Concatenate Strings(w431, "\\\\" ("format string"), w426, "_" ("format string"), w417, w416) -> (w430:string)
                n262 = String To Path(string=w430) -> (path=w429:path)
                n263 = call <vilib>:"Check if File or Folder Exists.vi"("path"=w429) -> ("dup path"=w422:path)  [unwired: 8 in, 2 out]
                n264 = case shown="True" TRUE {
                  tunnel: w422 -> [w435 w437]
                  tunnel: [w436 w437] -> _
                  frame False {
                    n265 = Create Folder(path (use dialog)=w435) -> (created path=w436:path)  [unwired: 2 in, 2 out]
                  }
                  frame True {
                  }
                }
                n266 = local write "fileName"(w422) -> ()
              }
              frame #1 {
                n267 = local read "FIB/SEM"() -> (w439:bool)
                n268 = case shown="False" w439 {
                  tunnel: ["_FIB" ("format string") "_SEM" ("format string")] -> w438
                  frame False {
                  }
                  frame True {
                  }
                }
                n269 = TCP Open Connection(address="localhost", remote port or service name=u16 8089) -> (connection ID=w445:refnum<k5>, error out=w444:errorcluster)  [unwired: 3 in]
                n270 = TCP Write(connection ID=w445, data in=w438, error in (no error)=w444) -> (connection ID out=w450:refnum<k5>, error out=w449:errorcluster)  [unwired: 1 in, 1 out]
                n271 = TCP Read(connection ID=w450, bytes to read=9, error in (no error)=w449, 9:20000 ("timeout ms (25000)")) -> (connection ID out=w443:refnum<k5>, data out=w440:string, error out=w442:errorcluster)  [unwired: 1 in]
                n272 = TCP Close Connection(connection ID=w443, error in (no error)=w442) -> ()  [unwired: 1 in, 2 out]
                n273 = local write "data out"(w440) -> ()
              }
              frame #2 {
                n274 = flat-sequence {
                  frame #0 {
                    n275 = TCP Open Connection(address="localhost", remote port or service name=u16 8089) -> (connection ID=w458:refnum<k5>, error out=w457:errorcluster)  [unwired: 3 in]
                    n276 = TCP Write(connection ID=w458, data in="DWEL", error in (no error)=w457) -> (connection ID out=w463:refnum<k5>, error out=w462:errorcluster)  [unwired: 1 in, 1 out]
                    n277 = TCP Read(connection ID=w463, bytes to read=9, error in (no error)=w462, 9:20000 ("timeout ms (25000)")) -> (connection ID out=w456:refnum<k5>, data out=w453:string, error out=w455:errorcluster)  [unwired: 1 in]
                    n278 = local write "data out"(w453) -> ()
                    n279 = TCP Close Connection(connection ID=w456, error in (no error)=w455) -> ()  [unwired: 1 in, 2 out]
                  }
                  frame #1 {
                    n280 = local read "Dwell time us"() -> (w477:dbl)
                    n281 = TCP Open Connection(address="localhost", remote port or service name=u16 8089) -> (connection ID=w471:refnum<k5>, error out=w472:errorcluster)  [unwired: 3 in]
                    n282 = Format Into String(format string=" %1.2f", initial string="", w477) -> (resulting string=w465:string)  [unwired: 1 in, 1 out]
                    n283 = TCP Write(connection ID=w471, data in=w465, error in (no error)=w472) -> (connection ID out=w466:refnum<k5>, error out=w467:errorcluster)  [unwired: 1 in, 1 out]
                    n284 = TCP Read(connection ID=w466, bytes to read=9, error in (no error)=w467, 9:20000 ("timeout ms (25000)")) -> (connection ID out=w473:refnum<k5>, data out=w476:string, error out=w474:errorcluster)  [unwired: 1 in]
                    n285 = local write "data out"(w476) -> ()
                    n286 = TCP Close Connection(connection ID=w473, error in (no error)=w474) -> ()  [unwired: 1 in, 2 out]
                  }
                }
              }
              frame #3 {
                n287 = flat-sequence {
                  frame #0 {
                    n288 = TCP Open Connection(address="localhost", remote port or service name=u16 8089) -> (connection ID=w485:refnum<k5>, error out=w484:errorcluster)  [unwired: 3 in]
                    n289 = TCP Write(connection ID=w485, data in="_DIR", error in (no error)=w484) -> (connection ID out=w490:refnum<k5>, error out=w489:errorcluster)  [unwired: 1 in, 1 out]
                    n290 = TCP Read(connection ID=w490, bytes to read=9, error in (no error)=w489, 9:20000 ("timeout ms (25000)")) -> (connection ID out=w483:refnum<k5>, data out=w480:string, error out=w482:errorcluster)  [unwired: 1 in]
                    n291 = local write "data out"(w480) -> ()
                    n292 = TCP Close Connection(connection ID=w483, error in (no error)=w482) -> ()  [unwired: 1 in, 2 out]
                  }
                  frame #1 {
                    n293 = local read "fileName"() -> (w496:path)
                    n294 = Path To String(path=w496) -> (string=w494:string)
                    n295 = TCP Open Connection(address="localhost", remote port or service name=u16 8089) -> (connection ID=w502:refnum<k5>, error out=w503:errorcluster)  [unwired: 3 in]
                    n296 = Format Into String(format string=" %1028s", initial string=w494, "") -> (resulting string=w495:string)  [unwired: 1 in, 1 out]
                    n297 = TCP Write(connection ID=w502, data in=w495, error in (no error)=w503) -> (connection ID out=w497:refnum<k5>, error out=w498:errorcluster)  [unwired: 1 in, 1 out]
                    n298 = TCP Read(connection ID=w497, bytes to read=9, error in (no error)=w498, 9:20000 ("timeout ms (25000)")) -> (connection ID out=w504:refnum<k5>, data out=w507:string, error out=w505:errorcluster)  [unwired: 1 in]
                    n299 = local write "data out"(w507) -> ()
                    n300 = TCP Close Connection(connection ID=w504, error in (no error)=w505) -> ()  [unwired: 1 in, 2 out]
                  }
                }
              }
              frame #4 {
                n301 = TCP Open Connection(address="localhost", remote port or service name=u16 8089) -> (connection ID=w513:refnum<k5>, error out=w512:errorcluster)  [unwired: 3 in]
                n302 = TCP Write(connection ID=w513, data in="IMGS", error in (no error)=w512) -> (connection ID out=w518:refnum<k5>, error out=w517:errorcluster)  [unwired: 1 in, 1 out]
                n303 = TCP Read(connection ID=w518, bytes to read=9, error in (no error)=w517, 9:20000 ("timeout ms (25000)")) -> (connection ID out=w511:refnum<k5>, data out=w508:string, error out=w510:errorcluster)  [unwired: 1 in]
                n304 = TCP Close Connection(connection ID=w511, error in (no error)=w510) -> ()  [unwired: 1 in, 2 out]
                n305 = local write "data out"(w508) -> ()
              }
              frame #5 {
                n306 = TCP Open Connection(address="localhost", remote port or service name=u16 8089) -> (connection ID=w526:refnum<k5>, error out=w525:errorcluster)  [unwired: 3 in]
                n307 = TCP Write(connection ID=w526, data in="GETL", error in (no error)=w525) -> (connection ID out=w531:refnum<k5>, error out=w530:errorcluster)  [unwired: 1 in, 1 out]
                n308 = TCP Read(connection ID=w531, bytes to read=20, error in (no error)=w530, 9:5000 ("timeout ms (25000)")) -> (connection ID out=w524:refnum<k5>, data out=w521:string, error out=w523:errorcluster)  [unwired: 1 in]
                n309 = Decimal String To Number(string=w521) -> (number=w520:i32)  [unwired: 2 in, 1 out]
                n310 = local write "data out"(w521) -> ()
                n311 = local write "length"(w520) -> ()
                n312 = TCP Close Connection(connection ID=w524, error in (no error)=w523) -> ()  [unwired: 1 in, 2 out]
              }
              frame #6 {
                n313 = property on="Grab FIB-SEM OLD" class="Bool (strict)"("Value"=FALSE ("Grab Image")) -> ()  [unwired: 2 in, 2 out]
                n314 = TCP Open Connection(address="localhost", remote port or service name=u16 8089) -> (connection ID=w549:refnum<k5>, error out=w550:errorcluster)  [unwired: 3 in]
                n315 = local read "length"() -> (w551:i32)
                n316 = TCP Write(connection ID=w549, data in="DATA", error in (no error)=w550) -> (connection ID out=w544:refnum<k5>, error out=w545:errorcluster)  [unwired: 1 in, 1 out]
                n317 = TCP Read(connection ID=w544, bytes to read=w551, error in (no error)=w545, 9:5000 ("timeout ms (25000)")) -> (data out=w534:string)  [unwired: 1 in, 2 out]
                n318 = Spreadsheet String To Array(delimiter (Tab)=" ", format string="", spreadsheet string=w534) -> (array=w540:dbl[][])  [unwired: 1 in]
                n319 = local read "xc"() -> (w535:i32)
                n320 = local read "yc"() -> (w536:i32)
                n321 = To Long Integer(number=w540) -> (32bit integer=w539:i32[][])
                n322 = Reshape Array(w539, w535, w536) -> (w541:i32[][])
                n323 = To Long Integer(number=w541) -> (32bit integer=w542:i32[][])
                n324 = local write "Intensity FIB-SEM"(w542) -> ()
              }
              frame #7 {
                # "what is the length of the data - PATH?"
                n325 = property on="Grab FIB-SEM" class="Bool (strict)"("Value"=FALSE ("Grab FIB-SEM TCP")) -> ()  [unwired: 2 in, 2 out]
                n326 = TCP Open Connection(address="localhost", remote port or service name=u16 8089) -> (connection ID=w558:refnum<k5>, error out=w557:errorcluster)  [unwired: 3 in]
                n327 = TCP Write(connection ID=w558, data in="GLPT", error in (no error)=w557) -> (connection ID out=w563:refnum<k5>, error out=w562:errorcluster)  [unwired: 1 in, 1 out]
                n328 = TCP Read(connection ID=w563, bytes to read=20, error in (no error)=w562, 9:5000 ("timeout ms (25000)")) -> (connection ID out=w556:refnum<k5>, data out=w553:string, error out=w555:errorcluster)  [unwired: 1 in]
                n329 = Decimal String To Number(string=w553) -> (number=w552:i32)  [unwired: 2 in, 1 out]
                n330 = local write "data out"(w553) -> ()
                n331 = TCP Close Connection(connection ID=w556, error in (no error)=w555) -> ()  [unwired: 1 in, 2 out]
                n332 = local write "length"(w552) -> ()
              }
              frame #8 {
                # "file path to the merged bmp"
                n333 = TCP Open Connection(address="localhost", remote port or service name=u16 8089) -> (connection ID=w574:refnum<k5>, error out=w575:errorcluster)  [unwired: 3 in]
                n334 = local read "length"() -> (w576:i32)
                n335 = TCP Write(connection ID=w574, data in="DTPH", error in (no error)=w575) -> (connection ID out=w569:refnum<k5>, error out=w570:errorcluster)  [unwired: 1 in, 1 out]
                n336 = TCP Read(connection ID=w569, bytes to read=w576, error in (no error)=w570, 9:5000 ("timeout ms (25000)")) -> (data out=w567:string)  [unwired: 1 in, 2 out]
                n337 = String To Path(string=w567) -> (path=w566:path)
                n338 = local write "pythonOut"(w567) -> ()
                n339 = local write "fileNameFIBSEM"(w566) -> ()
              }
            }
          }
          event "Grab Image": Value Change {
            n340 = event-data() -> ()  [unwired: 1 in, 6 out]
            n341 = stacked-sequence {
              tunnel: w577 -> [w582 _ _ _ _ _ _ _]
              frame #0 {
                w578 = "_" ("format string")
                n342 = local read "lambda"() -> (w586:dbl)
                n343 = local read "Path"() -> (w591:path)
                n344 = local read "File Prefix"() -> (w589:string)
                n345 = Number To Decimal String(number=w586) -> (decimal integer string=w579:string)  [unwired: 1 in]
                n346 = Increment(x=w582) -> (x+1=w583:i32)
                n347 = Path To String(path=w591) -> (string=w594:string)
                n348 = Format Into String(format string="%03d", w583) -> (resulting string=w581:string)  [unwired: 2 in, 1 out]
                n349 = Format Date/Time String(time format string (%c)="%Y_%m_%d_%H_%M_%S") -> (date/time string=w585:string)  [unwired: 2 in]
                n350 = local write "date/time string"(w585) -> ()
                n351 = Concatenate Strings(w594, "\\\\" ("format string"), w589, w578, w581, "_OPT_" ("format string"), w579, w578) -> (w593:string)
                n352 = String To Path(string=w593) -> (path=w592:path)
                n353 = call <vilib>:"Check if File or Folder Exists.vi"("path"=w592) -> ("dup path"=w587:path)  [unwired: 8 in, 2 out]
                n354 = case shown="True" TRUE {
                  tunnel: w587 -> [w596 w598]
                  tunnel: [w597 w598] -> _
                  frame False {
                    n355 = Create Folder(path (use dialog)=w596) -> (created path=w597:path)  [unwired: 2 in, 2 out]
                  }
                  frame True {
                  }
                }
                n356 = local write "fileName"(w587) -> ()
              }
              frame #1 {
                n357 = TCP Open Connection(address="localhost", remote port or service name=u16 8089) -> (connection ID=w605:refnum<k5>, error out=w604:errorcluster)  [unwired: 3 in]
                n358 = TCP Write(connection ID=w605, data in="_OPT" ("format string"), error in (no error)=w604) -> (connection ID out=w610:refnum<k5>, error out=w609:errorcluster)  [unwired: 1 in, 1 out]
                n359 = TCP Read(connection ID=w610, bytes to read=9, error in (no error)=w609, 9:20000 ("timeout ms (25000)")) -> (connection ID out=w603:refnum<k5>, data out=w600:string, error out=w602:errorcluster)  [unwired: 1 in]
                n360 = TCP Close Connection(connection ID=w603, error in (no error)=w602) -> ()  [unwired: 1 in, 2 out]
                n361 = local write "data out"(w600) -> ()
              }
              frame #2 {
                n362 = flat-sequence {
                  frame #0 {
                    n363 = TCP Open Connection(address="localhost", remote port or service name=u16 8089) -> (connection ID=w616:refnum<k5>, error out=w615:errorcluster)  [unwired: 3 in]
                    n364 = TCP Write(connection ID=w616, data in="EXPS", error in (no error)=w615) -> (connection ID out=w621:refnum<k5>, error out=w620:errorcluster)  [unwired: 1 in, 1 out]
                    n365 = TCP Read(connection ID=w621, bytes to read=9, error in (no error)=w620, 9:20000 ("timeout ms (25000)")) -> (connection ID out=w614:refnum<k5>, data out=w611:string, error out=w613:errorcluster)  [unwired: 1 in]
                    n366 = local write "data out"(w611) -> ()
                    n367 = TCP Close Connection(connection ID=w614, error in (no error)=w613) -> ()  [unwired: 1 in, 2 out]
                  }
                  frame #1 {
                    n368 = local read "Exposure ms"() -> (w625:i32)
                    n369 = TCP Open Connection(address="localhost", remote port or service name=u16 8089) -> (connection ID=w632:refnum<k5>, error out=w633:errorcluster)  [unwired: 3 in]
                    n370 = Number To Decimal String(number=w625) -> (decimal integer string=w624:string)  [unwired: 1 in]
                    n371 = Format Into String(format string=" %4s", initial string=w624, "") -> (resulting string=w626:string)  [unwired: 1 in, 1 out]
                    n372 = TCP Write(connection ID=w632, data in=w626, error in (no error)=w633) -> (connection ID out=w627:refnum<k5>, error out=w628:errorcluster)  [unwired: 1 in, 1 out]
                    n373 = TCP Read(connection ID=w627, bytes to read=9, error in (no error)=w628, 9:20000 ("timeout ms (25000)")) -> (connection ID out=w634:refnum<k5>, data out=w637:string, error out=w635:errorcluster)  [unwired: 1 in]
                    n374 = local write "data out"(w637) -> ()
                    n375 = TCP Close Connection(connection ID=w634, error in (no error)=w635) -> ()  [unwired: 1 in, 2 out]
                  }
                }
              }
              frame #3 {
                n376 = flat-sequence {
                  frame #0 {
                    n377 = TCP Open Connection(address="localhost", remote port or service name=u16 8089) -> (connection ID=w644:refnum<k5>, error out=w643:errorcluster)  [unwired: 3 in]
                    n378 = TCP Write(connection ID=w644, data in="_DIR", error in (no error)=w643) -> (connection ID out=w649:refnum<k5>, error out=w648:errorcluster)  [unwired: 1 in, 1 out]
                    n379 = TCP Read(connection ID=w649, bytes to read=9, error in (no error)=w648, 9:20000 ("timeout ms (25000)")) -> (connection ID out=w642:refnum<k5>, data out=w639:string, error out=w641:errorcluster)  [unwired: 1 in]
                    n380 = local write "data out"(w639) -> ()
                    n381 = TCP Close Connection(connection ID=w642, error in (no error)=w641) -> ()  [unwired: 1 in, 2 out]
                  }
                  frame #1 {
                    n382 = local read "fileName"() -> (w655:path)
                    n383 = Path To String(path=w655) -> (string=w653:string)
                    n384 = TCP Open Connection(address="localhost", remote port or service name=u16 8089) -> (connection ID=w661:refnum<k5>, error out=w662:errorcluster)  [unwired: 3 in]
                    n385 = Format Into String(format string=" %1028s", initial string=w653, "") -> (resulting string=w654:string)  [unwired: 1 in, 1 out]
                    n386 = TCP Write(connection ID=w661, data in=w654, error in (no error)=w662) -> (connection ID out=w656:refnum<k5>, error out=w657:errorcluster)  [unwired: 1 in, 1 out]
                    n387 = TCP Read(connection ID=w656, bytes to read=9, error in (no error)=w657, 9:20000 ("timeout ms (25000)")) -> (connection ID out=w663:refnum<k5>, data out=w666:string, error out=w664:errorcluster)  [unwired: 1 in]
                    n388 = local write "data out"(w666) -> ()
                    n389 = TCP Close Connection(connection ID=w663, error in (no error)=w664) -> ()  [unwired: 1 in, 2 out]
                  }
                }
              }
              frame #4 {
                n390 = TCP Open Connection(address="localhost", remote port or service name=u16 8089) -> (connection ID=w672:refnum<k5>, error out=w671:errorcluster)  [unwired: 3 in]
                n391 = TCP Write(connection ID=w672, data in="IMGO", error in (no error)=w671) -> (connection ID out=w677:refnum<k5>, error out=w676:errorcluster)  [unwired: 1 in, 1 out]
                n392 = TCP Read(connection ID=w677, bytes to read=9, error in (no error)=w676, 9:20000 ("timeout ms (25000)")) -> (connection ID out=w670:refnum<k5>, data out=w667:string, error out=w669:errorcluster)  [unwired: 1 in]
                n393 = TCP Close Connection(connection ID=w670, error in (no error)=w669) -> ()  [unwired: 1 in, 2 out]
                n394 = local write "data out"(w667) -> ()
              }
              frame #5 {
                n395 = TCP Open Connection(address="localhost", remote port or service name=u16 8089) -> (connection ID=w685:refnum<k5>, error out=w684:errorcluster)  [unwired: 3 in]
                n396 = TCP Write(connection ID=w685, data in="GETL", error in (no error)=w684) -> (connection ID out=w690:refnum<k5>, error out=w689:errorcluster)  [unwired: 1 in, 1 out]
                n397 = TCP Read(connection ID=w690, bytes to read=20, error in (no error)=w689, 9:5000 ("timeout ms (25000)")) -> (connection ID out=w683:refnum<k5>, data out=w680:string, error out=w682:errorcluster)  [unwired: 1 in]
                n398 = Decimal String To Number(string=w680) -> (number=w679:i32)  [unwired: 2 in, 1 out]
                n399 = local write "data out"(w680) -> ()
                n400 = TCP Close Connection(connection ID=w683, error in (no error)=w682) -> ()  [unwired: 1 in, 2 out]
                n401 = local write "length"(w679) -> ()
              }
              frame #6 {
                n402 = property on="Grab Image" class="Bool (strict)"("Value"=FALSE ("Grab Image TCP")) -> ()  [unwired: 2 in, 2 out]
                n403 = TCP Open Connection(address="localhost", remote port or service name=u16 8089) -> (connection ID=w708:refnum<k5>, error out=w709:errorcluster)  [unwired: 3 in]
                n404 = local read "length"() -> (w710:i32)
                n405 = TCP Write(connection ID=w708, data in="DATA", error in (no error)=w709) -> (connection ID out=w703:refnum<k5>, error out=w704:errorcluster)  [unwired: 1 in, 1 out]
                n406 = TCP Read(connection ID=w703, bytes to read=w710, error in (no error)=w704, 9:5000 ("timeout ms (25000)")) -> (data out=w693:string)  [unwired: 1 in, 2 out]
                n407 = Spreadsheet String To Array(delimiter (Tab)=" ", format string="", spreadsheet string=w693) -> (array=w699:dbl[][])  [unwired: 1 in]
                n408 = local read "yo"() -> (w694:i32)
                n409 = local read "xo"() -> (w695:i32)
                n410 = To Long Integer(number=w699) -> (32bit integer=w698:i32[][])
                n411 = Reshape Array(w698, w694, w695) -> (w700:i32[][])
                n412 = To Long Integer(number=w700) -> (32bit integer=w701:i32[][])
                n413 = local write "Intensity OPT"(w701) -> ()
              }
              frame #7 {
                n414 = TCP Open Connection(address="localhost", remote port or service name=u16 8089) -> (connection ID=w715:refnum<k5>, error out=w714:errorcluster)  [unwired: 3 in]
                n415 = TCP Write(connection ID=w715, data in="QUI_", error in (no error)=w714) -> (connection ID out=w720:refnum<k5>, error out=w719:errorcluster)  [unwired: 1 in, 1 out]
                n416 = TCP Read(connection ID=w720, bytes to read=9, error in (no error)=w719, 9:5000 ("timeout ms (25000)")) -> (connection ID out=w713:refnum<k5>, data out=w711:string, error out=w712:errorcluster)  [unwired: 1 in]
                n417 = local write "done"(w711) -> ()
                n418 = TCP Close Connection(connection ID=w713, error in (no error)=w712) -> ()  [unwired: 1 in, 2 out]
              }
            }
          }
          event "Two lambda grab OLD": Value Change {
            n419 = event-data() -> ()  [unwired: 1 in, 6 out]
            n420 = stacked-sequence {
              frame #0 {
                # "Initialise the first laser, get the lambda"
                n421 = local read "baud rate Obis"() -> (w737:u32)
                n422 = call "sub - Laser Get WaveLength.vi"("VISA resource name"=refnum<visa-resource-name> "COM11", "baud rate (9600)"=w737) -> ("reference out"=w726:refnum<visa-resource-name>, "wavelength"=w729:dbl, "error out"=w742:errorcluster, "message"=w743:string)  [unwired: 1 in, 1 out]
                n423 = call "sub - Laser Get Power Limits.vi"("VISA resource name"=w726, "baud rate (9600)"=w737, "error in (no error)"=w742) -> ("powerNominal"=w735:dbl, "powerMin"=w741:dbl, "powerMax"=w740:dbl, "error out"=w739:errorcluster)  [unwired: 1 out]
                n424 = local write "lambda"(w729) -> ()
                n425 = call "sub - Laser Get Power.vi"("VISA resource name"=w726, "baud rate (9600)"=w737, "error in (no error)"=w739) -> ("reference out"=w724:refnum<visa-resource-name>, "Power"=w736:dbl, "error out"=w738:errorcluster)  [unwired: 2 out]
                n426 = Format Into String(format string="%d", w729) -> (resulting string=w725:string)  [unwired: 2 in, 1 out]
                n427 = local write "Power1max"(w740) -> ()
                n428 = local write "PowerNom1"(w735) -> ()
                n429 = local write "Power1min"(w741) -> ()
                n430 = local write "error Obis"(w738) -> ()
                n431 = local write "Message Obis"(w743) -> ()
                n432 = local write "Power"(w736) -> ()
                n433 = Concatenate Strings("wav" ("string"), w725) -> (w727:string)
                n434 = local write "wav 1"(w727) -> ()
                n435 = Divide(x=w736, y=w735) -> (x/y=w734:dbl)
                n436 = local write "Obis out"(w724) -> ()
                n437 = Multiply(x=w734, y=100.0) -> (x*y=w731:dbl)
                n438 = To Long Integer(number=w731) -> (32bit integer=w732:i32)
                n439 = local write "Power L1 %"(w732) -> ()
              }
              frame #1 {
                w744 = "_" ("format string")
                # "Make the directory name with the wavelength"
                n440 = local read "lambda"() -> (w748:dbl)
                n441 = local read "Path"() -> (w753:path)
                n442 = Path To String(path=w753) -> (string=w756:string)
                n443 = local read "DIR Series"() -> (w749:string)
                n444 = Number To Decimal String(number=w748) -> (decimal integer string=w747:string)  [unwired: 1 in]
                n445 = Format Date/Time String(time format string (%c)="%Y_%m_%d_%H_%M_%S") -> (date/time string=w745:string)  [unwired: 2 in]
                n446 = Concatenate Strings(w756, "\\\\" ("format string"), w749, w747, w744, "_OPT_" ("format string"), w745, w744) -> (w755:string)
                n447 = local write "date/time string"(w745) -> ()
                n448 = String To Path(string=w755) -> (path=w754:path)
                n449 = call <vilib>:"Check if File or Folder Exists.vi"("path"=w754) -> ("file or folder exists?"=w752:bool, "dup path"=w751:path)  [unwired: 8 in, 1 out]
                n450 = case shown="False" w752 {
                  tunnel: w751 -> [w759 w761]
                  tunnel: [w760 w761] -> w758
                  frame False {
                    n451 = Create Folder(path (use dialog)=w759) -> (created path=w760:path)  [unwired: 2 in, 2 out]
                  }
                  frame True {
                  }
                }
                n452 = local write "Path series"(w758) -> ()
              }
              frame #2 {
                n453 = TCP Open Connection(address="localhost", remote port or service name=u16 8089) -> (connection ID=w768:refnum<k5>, error out=w767:errorcluster)  [unwired: 3 in]
                n454 = TCP Write(connection ID=w768, data in="_OPT" ("format string"), error in (no error)=w767) -> (connection ID out=w773:refnum<k5>, error out=w772:errorcluster)  [unwired: 1 in, 1 out]
                n455 = TCP Read(connection ID=w773, bytes to read=9, error in (no error)=w772, 9:20000 ("timeout ms (25000)")) -> (connection ID out=w766:refnum<k5>, data out=w763:string, error out=w765:errorcluster)  [unwired: 1 in]
                n456 = TCP Close Connection(connection ID=w766, error in (no error)=w765) -> ()  [unwired: 1 in, 2 out]
                n457 = local write "data out"(w763) -> ()
              }
              frame #3 {
                n458 = flat-sequence {
                  frame #0 {
                    n459 = TCP Open Connection(address="localhost", remote port or service name=u16 8089) -> (connection ID=w779:refnum<k5>, error out=w778:errorcluster)  [unwired: 3 in]
                    n460 = TCP Write(connection ID=w779, data in="EXPS", error in (no error)=w778) -> (connection ID out=w784:refnum<k5>, error out=w783:errorcluster)  [unwired: 1 in, 1 out]
                    n461 = TCP Read(connection ID=w784, bytes to read=9, error in (no error)=w783, 9:20000 ("timeout ms (25000)")) -> (connection ID out=w777:refnum<k5>, data out=w774:string, error out=w776:errorcluster)  [unwired: 1 in]
                    n462 = local write "data out"(w774) -> ()
                    n463 = TCP Close Connection(connection ID=w777, error in (no error)=w776) -> ()  [unwired: 1 in, 2 out]
                  }
                  frame #1 {
                    n464 = local read "Exposure ms"() -> (w788:i32)
                    n465 = TCP Open Connection(address="localhost", remote port or service name=u16 8089) -> (connection ID=w795:refnum<k5>, error out=w796:errorcluster)  [unwired: 3 in]
                    n466 = Number To Decimal String(number=w788) -> (decimal integer string=w787:string)  [unwired: 1 in]
                    n467 = Format Into String(format string=" %4s", initial string=w787, "") -> (resulting string=w789:string)  [unwired: 1 in, 1 out]
                    n468 = TCP Write(connection ID=w795, data in=w789, error in (no error)=w796) -> (connection ID out=w790:refnum<k5>, error out=w791:errorcluster)  [unwired: 1 in, 1 out]
                    n469 = TCP Read(connection ID=w790, bytes to read=9, error in (no error)=w791, 9:20000 ("timeout ms (25000)")) -> (connection ID out=w797:refnum<k5>, data out=w800:string, error out=w798:errorcluster)  [unwired: 1 in]
                    n470 = local write "data out"(w800) -> ()
                    n471 = TCP Close Connection(connection ID=w797, error in (no error)=w798) -> ()  [unwired: 1 in, 2 out]
                  }
                }
              }
              frame #4 {
                n472 = flat-sequence {
                  frame #0 {
                    n473 = TCP Open Connection(address="localhost", remote port or service name=u16 8089) -> (connection ID=w807:refnum<k5>, error out=w806:errorcluster)  [unwired: 3 in]
                    n474 = TCP Write(connection ID=w807, data in="_DIR", error in (no error)=w806) -> (connection ID out=w812:refnum<k5>, error out=w811:errorcluster)  [unwired: 1 in, 1 out]
                    n475 = TCP Read(connection ID=w812, bytes to read=9, error in (no error)=w811, 9:20000 ("timeout ms (25000)")) -> (connection ID out=w805:refnum<k5>, data out=w802:string, error out=w804:errorcluster)  [unwired: 1 in]
                    n476 = local write "data out"(w802) -> ()
                    n477 = TCP Close Connection(connection ID=w805, error in (no error)=w804) -> ()  [unwired: 1 in, 2 out]
                  }
                  frame #1 {
                    n478 = local read "Path series"() -> (w818:path)
                    n479 = Path To String(path=w818) -> (string=w816:string)
                    n480 = TCP Open Connection(address="localhost", remote port or service name=u16 8089) -> (connection ID=w824:refnum<k5>, error out=w825:errorcluster)  [unwired: 3 in]
                    n481 = Format Into String(format string=" %1028s", initial string=w816, "") -> (resulting string=w817:string)  [unwired: 1 in, 1 out]
                    n482 = TCP Write(connection ID=w824, data in=w817, error in (no error)=w825) -> (connection ID out=w819:refnum<k5>, error out=w820:errorcluster)  [unwired: 1 in, 1 out]
                    n483 = TCP Read(connection ID=w819, bytes to read=9, error in (no error)=w820, 9:20000 ("timeout ms (25000)")) -> (connection ID out=w826:refnum<k5>, data out=w829:string, error out=w827:errorcluster)  [unwired: 1 in]
                    n484 = local write "data out"(w829) -> ()
                    n485 = TCP Close Connection(connection ID=w826, error in (no error)=w827) -> ()  [unwired: 1 in, 2 out]
                  }
                }
              }
              frame #5 {
                # "LASER ON"
                n486 = local read "baud rate Obis"() -> (w839:u32)
                n487 = local read "error Obis"() -> (w832:errorcluster)
                n488 = call "sub - Laser ON or OFF.vi"("error in (no error)"=w832, "ON/OFF"=TRUE, "baud rate (9600)"=w839, "VISA resource name"=refnum<visa-resource-name> "COM11") -> ("error out"=w840:errorcluster, "message"=w835:string, "reference out"=w838:refnum<visa-resource-name>)  [unwired: 1 out]
                n489 = String Subset(string=w835, length (rest)=2 ("length (rest)")) -> (substring=w837:string)  [unwired: 1 in]
                n490 = Equal?(x=w837, y="OK") -> (x = y?=w834:bool)
                n491 = local write "Message Obis"(w835) -> ()
                n492 = local write "error Obis"(w840) -> ()
                n493 = case shown="True" w834 {
                  tunnel: w838 -> [_ w845]
                  tunnel: w840 -> [_ w848]
                  tunnel: w839 -> [_ w843]
                  frame False {
                    n494 = local write "Obis"(FALSE ("Obis")) -> ()
                  }
                  frame True {
                    n495 = call "sub - Laser Get Status ON or OFF.vi"("VISA resource name"=w845, "baud rate (9600)"=w843, "error in (no error)"=w848) -> ("reference out"=w844:refnum<visa-resource-name>, "ON/OFF"=w847:bool, "message"=w846:string, "error out"=w842:errorcluster)  [unwired: 1 out]
                    n496 = local write "Message Obis"(w846) -> ()
                    n497 = local write "error Obis"(w842) -> ()
                    n498 = local write "Obis out"(w844) -> ()
                    n499 = local write "L1"(w847) -> ()
                  }
                }
              }
              frame #6 {
                # "Take a shot"
                n500 = TCP Open Connection(address="localhost", remote port or service name=u16 8089) -> (connection ID=w854:refnum<k5>, error out=w853:errorcluster)  [unwired: 3 in]
                n501 = TCP Write(connection ID=w854, data in="IMGO", error in (no error)=w853) -> (connection ID out=w859:refnum<k5>, error out=w858:errorcluster)  [unwired: 1 in, 1 out]
                n502 = TCP Read(connection ID=w859, bytes to read=9, error in (no error)=w858, 9:20000 ("timeout ms (25000)")) -> (connection ID out=w852:refnum<k5>, data out=w849:string, error out=w851:errorcluster)  [unwired: 1 in]
                n503 = TCP Close Connection(connection ID=w852, error in (no error)=w851) -> ()  [unwired: 1 in, 2 out]
                n504 = local write "data out"(w849) -> ()
              }
              frame #7 {
                # "LASER OFF"
                n505 = local read "baud rate Obis"() -> (w870:u32)
                n506 = local read "error Obis"() -> (w863:errorcluster)
                n507 = call "sub - Laser ON or OFF.vi"("error in (no error)"=w863, "ON/OFF"=FALSE, "baud rate (9600)"=w870, "VISA resource name"=refnum<visa-resource-name> "COM11") -> ("error out"=w871:errorcluster, "message"=w866:string, "reference out"=w869:refnum<visa-resource-name>)  [unwired: 1 out]
                n508 = String Subset(string=w866, length (rest)=2 ("length (rest)")) -> (substring=w868:string)  [unwired: 1 in]
                n509 = Equal?(x=w868, y="OK") -> (x = y?=w865:bool)
                n510 = local write "Message Obis"(w866) -> ()
                n511 = local write "error Obis"(w871) -> ()
                n512 = case shown="True" w865 {
                  tunnel: w869 -> [_ w876]
                  tunnel: w871 -> [_ w879]
                  tunnel: w870 -> [_ w874]
                  frame False {
                    n513 = local write "Obis"(FALSE ("Obis")) -> ()
                  }
                  frame True {
                    n514 = call "sub - Laser Get Status ON or OFF.vi"("VISA resource name"=w876, "baud rate (9600)"=w874, "error in (no error)"=w879) -> ("reference out"=w875:refnum<visa-resource-name>, "ON/OFF"=w878:bool, "message"=w877:string, "error out"=w873:errorcluster)  [unwired: 1 out]
                    n515 = local write "Message Obis"(w877) -> ()
                    n516 = local write "error Obis"(w873) -> ()
                    n517 = local write "Obis out"(w875) -> ()
                    n518 = local write "L1"(w878) -> ()
                  }
                }
              }
              frame #8 {
                # "what is the length of the data?"
                n519 = TCP Open Connection(address="localhost", remote port or service name=u16 8089) -> (connection ID=w886:refnum<k5>, error out=w885:errorcluster)  [unwired: 3 in]
                n520 = TCP Write(connection ID=w886, data in="GETL", error in (no error)=w885) -> (connection ID out=w891:refnum<k5>, error out=w890:errorcluster)  [unwired: 1 in, 1 out]
                n521 = TCP Read(connection ID=w891, bytes to read=20, error in (no error)=w890, 9:5000 ("timeout ms (25000)")) -> (connection ID out=w884:refnum<k5>, data out=w881:string, error out=w883:errorcluster)  [unwired: 1 in]
                n522 = Decimal String To Number(string=w881) -> (number=w880:i32)  [unwired: 2 in, 1 out]
                n523 = local write "data out"(w881) -> ()
                n524 = TCP Close Connection(connection ID=w884, error in (no error)=w883) -> ()  [unwired: 1 in, 2 out]
                n525 = local write "length"(w880) -> ()
              }
              frame #9 {
                # "get the data, plot the data"
                n526 = TCP Open Connection(address="localhost", remote port or service name=u16 8089) -> (connection ID=w908:refnum<k5>, error out=w909:errorcluster)  [unwired: 3 in]
                n527 = local read "length"() -> (w910:i32)
                n528 = TCP Write(connection ID=w908, data in="DATA", error in (no error)=w909) -> (connection ID out=w903:refnum<k5>, error out=w904:errorcluster)  [unwired: 1 in, 1 out]
                n529 = TCP Read(connection ID=w903, bytes to read=w910, error in (no error)=w904, 9:5000 ("timeout ms (25000)")) -> (data out=w893:string)  [unwired: 1 in, 2 out]
                n530 = Spreadsheet String To Array(delimiter (Tab)=" ", format string="", spreadsheet string=w893) -> (array=w899:dbl[][])  [unwired: 1 in]
                n531 = local read "yo"() -> (w894:i32)
                n532 = local read "xo"() -> (w895:i32)
                n533 = To Long Integer(number=w899) -> (32bit integer=w898:i32[][])
                n534 = Reshape Array(w898, w894, w895) -> (w900:i32[][])
                n535 = To Long Integer(number=w900) -> (32bit integer=w901:i32[][])
                n536 = local write "Intensity OPT"(w901) -> ()
              }
              frame #10 {
                # "Initialise the second laser, get the lambda"
                n537 = local read "baud rate Obis"() -> (w925:u32)
                n538 = call "sub - Laser Get WaveLength.vi"("VISA resource name"=refnum<visa-resource-name> "COM12", "baud rate (9600)"=w925) -> ("reference out"=w914:refnum<visa-resource-name>, "wavelength"=w917:dbl, "error out"=w930:errorcluster, "message"=w931:string)  [unwired: 1 in, 1 out]
                n539 = call "sub - Laser Get Power Limits.vi"("VISA resource name"=w914, "baud rate (9600)"=w925, "error in (no error)"=w930) -> ("powerNominal"=w923:dbl, "powerMin"=w929:dbl, "powerMax"=w928:dbl, "error out"=w927:errorcluster)  [unwired: 1 out]
                n540 = local write "lambda"(w917) -> ()
                n541 = call "sub - Laser Get Power.vi"("VISA resource name"=w914, "baud rate (9600)"=w925, "error in (no error)"=w927) -> ("reference out"=w912:refnum<visa-resource-name>, "Power"=w924:dbl, "error out"=w926:errorcluster)  [unwired: 2 out]
                n542 = Format Into String(format string="%d", w917) -> (resulting string=w913:string)  [unwired: 2 in, 1 out]
                n543 = local write "Power1max"(w928) -> ()
                n544 = local write "PowerNom1"(w923) -> ()
                n545 = local write "Power1min"(w929) -> ()
                n546 = local write "error Obis"(w926) -> ()
                n547 = local write "Message Obis"(w931) -> ()
                n548 = local write "Power"(w924) -> ()
                n549 = Concatenate Strings("wav" ("string"), w913) -> (w915:string)
                n550 = local write "wav 1"(w915) -> ()
                n551 = Divide(x=w924, y=w923) -> (x/y=w922:dbl)
                n552 = local write "Obis out"(w912) -> ()
                n553 = Multiply(x=w922, y=100.0) -> (x*y=w919:dbl)
                n554 = To Long Integer(number=w919) -> (32bit integer=w920:i32)
                n555 = local write "Power L1 %"(w920) -> ()
              }
              frame #11 {
                w932 = "_" ("format string")
                # "Make the directory name with the wavelength"
                n556 = local read "lambda"() -> (w936:dbl)
                n557 = local read "Path"() -> (w941:path)
                n558 = Path To String(path=w941) -> (string=w944:string)
                n559 = local read "DIR Series"() -> (w937:string)
                n560 = Number To Decimal String(number=w936) -> (decimal integer string=w935:string)  [unwired: 1 in]
                n561 = Format Date/Time String(time format string (%c)="%Y_%m_%d_%H_%M_%S") -> (date/time string=w933:string)  [unwired: 2 in]
                n562 = Concatenate Strings(w944, "\\\\" ("format string"), w937, w935, w932, "_OPT_" ("format string"), w933, w932) -> (w943:string)
                n563 = local write "date/time string"(w933) -> ()
                n564 = String To Path(string=w943) -> (path=w942:path)
                n565 = call <vilib>:"Check if File or Folder Exists.vi"("path"=w942) -> ("file or folder exists?"=w940:bool, "dup path"=w939:path)  [unwired: 8 in, 1 out]
                n566 = case shown="False" w940 {
                  tunnel: w939 -> [w947 w949]
                  tunnel: [w948 w949] -> w946
                  frame False {
                    n567 = Create Folder(path (use dialog)=w947) -> (created path=w948:path)  [unwired: 2 in, 2 out]
                  }
                  frame True {
                  }
                }
                n568 = local write "Path series"(w946) -> ()
              }
              frame #12 {
                n569 = TCP Open Connection(address="localhost", remote port or service name=u16 8089) -> (connection ID=w956:refnum<k5>, error out=w955:errorcluster)  [unwired: 3 in]
                n570 = TCP Write(connection ID=w956, data in="_OPT" ("format string"), error in (no error)=w955) -> (connection ID out=w961:refnum<k5>, error out=w960:errorcluster)  [unwired: 1 in, 1 out]
                n571 = TCP Read(connection ID=w961, bytes to read=9, error in (no error)=w960, 9:20000 ("timeout ms (25000)")) -> (connection ID out=w954:refnum<k5>, data out=w951:string, error out=w953:errorcluster)  [unwired: 1 in]
                n572 = TCP Close Connection(connection ID=w954, error in (no error)=w953) -> ()  [unwired: 1 in, 2 out]
                n573 = local write "data out"(w951) -> ()
              }
              frame #13 {
                n574 = flat-sequence {
                  frame #0 {
                    n575 = TCP Open Connection(address="localhost", remote port or service name=u16 8089) -> (connection ID=w967:refnum<k5>, error out=w966:errorcluster)  [unwired: 3 in]
                    n576 = TCP Write(connection ID=w967, data in="EXPS", error in (no error)=w966) -> (connection ID out=w972:refnum<k5>, error out=w971:errorcluster)  [unwired: 1 in, 1 out]
                    n577 = TCP Read(connection ID=w972, bytes to read=9, error in (no error)=w971, 9:20000 ("timeout ms (25000)")) -> (connection ID out=w965:refnum<k5>, data out=w962:string, error out=w964:errorcluster)  [unwired: 1 in]
                    n578 = local write "data out"(w962) -> ()
                    n579 = TCP Close Connection(connection ID=w965, error in (no error)=w964) -> ()  [unwired: 1 in, 2 out]
                  }
                  frame #1 {
                    n580 = local read "Exposure ms"() -> (w976:i32)
                    n581 = TCP Open Connection(address="localhost", remote port or service name=u16 8089) -> (connection ID=w983:refnum<k5>, error out=w984:errorcluster)  [unwired: 3 in]
                    n582 = Number To Decimal String(number=w976) -> (decimal integer string=w975:string)  [unwired: 1 in]
                    n583 = Format Into String(format string=" %4s", initial string=w975, "") -> (resulting string=w977:string)  [unwired: 1 in, 1 out]
                    n584 = TCP Write(connection ID=w983, data in=w977, error in (no error)=w984) -> (connection ID out=w978:refnum<k5>, error out=w979:errorcluster)  [unwired: 1 in, 1 out]
                    n585 = TCP Read(connection ID=w978, bytes to read=9, error in (no error)=w979, 9:20000 ("timeout ms (25000)")) -> (connection ID out=w985:refnum<k5>, data out=w988:string, error out=w986:errorcluster)  [unwired: 1 in]
                    n586 = local write "data out"(w988) -> ()
                    n587 = TCP Close Connection(connection ID=w985, error in (no error)=w986) -> ()  [unwired: 1 in, 2 out]
                  }
                }
              }
              frame #14 {
                n588 = flat-sequence {
                  frame #0 {
                    n589 = TCP Open Connection(address="localhost", remote port or service name=u16 8089) -> (connection ID=w995:refnum<k5>, error out=w994:errorcluster)  [unwired: 3 in]
                    n590 = TCP Write(connection ID=w995, data in="_DIR", error in (no error)=w994) -> (connection ID out=w1000:refnum<k5>, error out=w999:errorcluster)  [unwired: 1 in, 1 out]
                    n591 = TCP Read(connection ID=w1000, bytes to read=9, error in (no error)=w999, 9:20000 ("timeout ms (25000)")) -> (connection ID out=w993:refnum<k5>, data out=w990:string, error out=w992:errorcluster)  [unwired: 1 in]
                    n592 = local write "data out"(w990) -> ()
                    n593 = TCP Close Connection(connection ID=w993, error in (no error)=w992) -> ()  [unwired: 1 in, 2 out]
                  }
                  frame #1 {
                    n594 = local read "Path series"() -> (w1006:path)
                    n595 = Path To String(path=w1006) -> (string=w1004:string)
                    n596 = TCP Open Connection(address="localhost", remote port or service name=u16 8089) -> (connection ID=w1012:refnum<k5>, error out=w1013:errorcluster)  [unwired: 3 in]
                    n597 = Format Into String(format string=" %1028s", initial string=w1004, "") -> (resulting string=w1005:string)  [unwired: 1 in, 1 out]
                    n598 = TCP Write(connection ID=w1012, data in=w1005, error in (no error)=w1013) -> (connection ID out=w1007:refnum<k5>, error out=w1008:errorcluster)  [unwired: 1 in, 1 out]
                    n599 = TCP Read(connection ID=w1007, bytes to read=9, error in (no error)=w1008, 9:20000 ("timeout ms (25000)")) -> (connection ID out=w1014:refnum<k5>, data out=w1017:string, error out=w1015:errorcluster)  [unwired: 1 in]
                    n600 = local write "data out"(w1017) -> ()
                    n601 = TCP Close Connection(connection ID=w1014, error in (no error)=w1015) -> ()  [unwired: 1 in, 2 out]
                  }
                }
              }
              frame #15 {
                # "LASER ON"
                n602 = local read "baud rate Obis"() -> (w1026:u32)
                n603 = local read "error Obis"() -> (w1019:errorcluster)
                n604 = call "sub - Laser ON or OFF.vi"("error in (no error)"=w1019, "ON/OFF"=TRUE, "baud rate (9600)"=w1026, "VISA resource name"=refnum<visa-resource-name> "COM12") -> ("error out"=w1027:errorcluster, "message"=w1022:string, "reference out"=w1025:refnum<visa-resource-name>)  [unwired: 1 out]
                n605 = String Subset(string=w1022, length (rest)=2 ("length (rest)")) -> (substring=w1024:string)  [unwired: 1 in]
                n606 = Equal?(x=w1024, y="OK") -> (x = y?=w1021:bool)
                n607 = local write "Message Obis"(w1022) -> ()
                n608 = local write "error Obis"(w1027) -> ()
                n609 = case shown="True" w1021 {
                  tunnel: w1025 -> [_ w1033]
                  tunnel: w1027 -> [_ w1036]
                  tunnel: w1026 -> [_ w1031]
                  frame False {
                    n610 = local write "Obis"(FALSE ("Obis")) -> ()
                  }
                  frame True {
                    n611 = call "sub - Laser Get Status ON or OFF.vi"("VISA resource name"=w1033, "baud rate (9600)"=w1031, "error in (no error)"=w1036) -> ("reference out"=w1032:refnum<visa-resource-name>, "ON/OFF"=w1035:bool, "message"=w1034:string, "error out"=w1030:errorcluster)  [unwired: 1 out]
                    n612 = local write "Message Obis"(w1034) -> ()
                    n613 = local write "error Obis"(w1030) -> ()
                    n614 = local write "Obis out"(w1032) -> ()
                    n615 = local write "L1"(w1035) -> ()
                  }
                }
              }
              frame #16 {
                # "Take a shot"
                n616 = TCP Open Connection(address="localhost", remote port or service name=u16 8089) -> (connection ID=w1042:refnum<k5>, error out=w1041:errorcluster)  [unwired: 3 in]
                n617 = TCP Write(connection ID=w1042, data in="IMGO", error in (no error)=w1041) -> (connection ID out=w1047:refnum<k5>, error out=w1046:errorcluster)  [unwired: 1 in, 1 out]
                n618 = TCP Read(connection ID=w1047, bytes to read=9, error in (no error)=w1046, 9:20000 ("timeout ms (25000)")) -> (connection ID out=w1040:refnum<k5>, data out=w1037:string, error out=w1039:errorcluster)  [unwired: 1 in]
                n619 = TCP Close Connection(connection ID=w1040, error in (no error)=w1039) -> ()  [unwired: 1 in, 2 out]
                n620 = local write "data out"(w1037) -> ()
              }
              frame #17 {
                # "LASER OFF"
                n621 = local read "baud rate Obis"() -> (w1057:u32)
                n622 = local read "error Obis"() -> (w1050:errorcluster)
                n623 = call "sub - Laser ON or OFF.vi"("error in (no error)"=w1050, "ON/OFF"=FALSE, "baud rate (9600)"=w1057, "VISA resource name"=refnum<visa-resource-name> "COM12") -> ("error out"=w1058:errorcluster, "message"=w1053:string, "reference out"=w1056:refnum<visa-resource-name>)  [unwired: 1 out]
                n624 = String Subset(string=w1053, length (rest)=2 ("length (rest)")) -> (substring=w1055:string)  [unwired: 1 in]
                n625 = Equal?(x=w1055, y="OK") -> (x = y?=w1052:bool)
                n626 = local write "Message Obis"(w1053) -> ()
                n627 = local write "error Obis"(w1058) -> ()
                n628 = case shown="True" w1052 {
                  tunnel: w1056 -> [_ w1064]
                  tunnel: w1058 -> [_ w1067]
                  tunnel: w1057 -> [_ w1062]
                  frame False {
                    n629 = local write "Obis"(FALSE ("Obis")) -> ()
                  }
                  frame True {
                    n630 = call "sub - Laser Get Status ON or OFF.vi"("VISA resource name"=w1064, "baud rate (9600)"=w1062, "error in (no error)"=w1067) -> ("reference out"=w1063:refnum<visa-resource-name>, "ON/OFF"=w1066:bool, "message"=w1065:string, "error out"=w1061:errorcluster)  [unwired: 1 out]
                    n631 = local write "Message Obis"(w1065) -> ()
                    n632 = local write "error Obis"(w1061) -> ()
                    n633 = local write "Obis out"(w1063) -> ()
                    n634 = local write "L1"(w1066) -> ()
                  }
                }
              }
              frame #18 {
                # "what is the length of the data?"
                n635 = TCP Open Connection(address="localhost", remote port or service name=u16 8089) -> (connection ID=w1074:refnum<k5>, error out=w1073:errorcluster)  [unwired: 3 in]
                n636 = TCP Write(connection ID=w1074, data in="GETL", error in (no error)=w1073) -> (connection ID out=w1079:refnum<k5>, error out=w1078:errorcluster)  [unwired: 1 in, 1 out]
                n637 = TCP Read(connection ID=w1079, bytes to read=20, error in (no error)=w1078, 9:5000 ("timeout ms (25000)")) -> (connection ID out=w1072:refnum<k5>, data out=w1069:string, error out=w1071:errorcluster)  [unwired: 1 in]
                n638 = Decimal String To Number(string=w1069) -> (number=w1068:i32)  [unwired: 2 in, 1 out]
                n639 = local write "data out"(w1069) -> ()
                n640 = TCP Close Connection(connection ID=w1072, error in (no error)=w1071) -> ()  [unwired: 1 in, 2 out]
                n641 = local write "length"(w1068) -> ()
              }
              frame #19 {
                # "get the data, plot the data"
                n642 = TCP Open Connection(address="localhost", remote port or service name=u16 8089) -> (connection ID=w1096:refnum<k5>, error out=w1097:errorcluster)  [unwired: 3 in]
                n643 = local read "length"() -> (w1098:i32)
                n644 = TCP Write(connection ID=w1096, data in="DATA", error in (no error)=w1097) -> (connection ID out=w1091:refnum<k5>, error out=w1092:errorcluster)  [unwired: 1 in, 1 out]
                n645 = TCP Read(connection ID=w1091, bytes to read=w1098, error in (no error)=w1092, 9:5000 ("timeout ms (25000)")) -> (data out=w1081:string)  [unwired: 1 in, 2 out]
                n646 = Spreadsheet String To Array(delimiter (Tab)=" ", format string="", spreadsheet string=w1081) -> (array=w1087:dbl[][])  [unwired: 1 in]
                n647 = local read "yo"() -> (w1082:i32)
                n648 = local read "xo"() -> (w1083:i32)
                n649 = To Long Integer(number=w1087) -> (32bit integer=w1086:i32[][])
                n650 = Reshape Array(w1086, w1082, w1083) -> (w1088:i32[][])
                n651 = To Long Integer(number=w1088) -> (32bit integer=w1089:i32[][])
                n652 = local write "Intensity OPT"(w1089) -> ()
              }
              frame #20 {
                n653 = property on="Two lambda grab OLD" class="Bool (strict)"("Value"=FALSE ("Two lambda grab")) -> ()  [unwired: 2 in, 2 out]
                n654 = TCP Open Connection(address="localhost", remote port or service name=u16 8089) -> (connection ID=w1104:refnum<k5>, error out=w1103:errorcluster)  [unwired: 3 in]
                n655 = TCP Write(connection ID=w1104, data in="QUI_", error in (no error)=w1103) -> (connection ID out=w1109:refnum<k5>, error out=w1108:errorcluster)  [unwired: 1 in, 1 out]
                n656 = TCP Read(connection ID=w1109, bytes to read=9, error in (no error)=w1108, 9:5000 ("timeout ms (25000)")) -> (connection ID out=w1102:refnum<k5>, data out=w1100:string, error out=w1101:errorcluster)  [unwired: 1 in]
                n657 = local write "done"(w1100) -> ()
                n658 = TCP Close Connection(connection ID=w1102, error in (no error)=w1101) -> ()  [unwired: 1 in, 2 out]
              }
            }
          }
          event "Two lambda old2": Value Change {
            n659 = event-data() -> ()  [unwired: 1 in, 6 out]
            n660 = stacked-sequence {
              tunnel: w1112 -> [_ w1114 _ _ _ _ _ _ _ _ _ w1275 _ _ _ _ _ _ _ _ _]
              frame #0 {
                # "Initialise the first laser, get the lambda"
                n661 = local write "lambda"(561.0 ("lambda")) -> ()
              }
              frame #1 {
                w1115 = "_" ("format string")
                # "Make the filoename  with the wavelength"
                n662 = local read "lambda"() -> (w1121:dbl)
                n663 = local read "Path"() -> (w1126:path)
                n664 = Increment(x=w1114) -> (x+1=w1119:i32)
                n665 = local read "File Prefix"() -> (w1124:string)
                n666 = Number To Decimal String(number=w1121) -> (decimal integer string=w1116:string)  [unwired: 1 in]
                n667 = Format Into String(format string="%03d", w1119) -> (resulting string=w1118:string)  [unwired: 2 in, 1 out]
                n668 = Path To String(path=w1126) -> (string=w1129:string)
                n669 = Format Date/Time String(time format string (%c)="%Y_%m_%d_%H_%M_%S") -> (date/time string=w1130:string)  [unwired: 2 in]
                n670 = local write "date/time string"(w1130) -> ()
                n671 = Concatenate Strings(w1129, "\\\\" ("format string"), w1124, w1115, w1118, "_2colour_" ("format string"), w1116, w1115) -> (w1128:string)
                n672 = String To Path(string=w1128) -> (path=w1127:path)
                n673 = call <vilib>:"Check if File or Folder Exists.vi"("path"=w1127) -> ("dup path"=w1122:path)  [unwired: 8 in, 2 out]
                n674 = case shown="True" TRUE {
                  tunnel: w1122 -> [w1132 w1134]
                  tunnel: [w1133 w1134] -> _
                  frame False {
                    n675 = Create Folder(path (use dialog)=w1132) -> (created path=w1133:path)  [unwired: 2 in, 2 out]
                  }
                  frame True {
                  }
                }
                n676 = local write "fileName"(w1122) -> ()
              }
              frame #2 {
                n677 = TCP Open Connection(address="localhost", remote port or service name=u16 8089) -> (connection ID=w1141:refnum<k5>, error out=w1140:errorcluster)  [unwired: 3 in]
                n678 = TCP Write(connection ID=w1141, data in="_OPT" ("format string"), error in (no error)=w1140) -> (connection ID out=w1146:refnum<k5>, error out=w1145:errorcluster)  [unwired: 1 in, 1 out]
                n679 = TCP Read(connection ID=w1146, bytes to read=9, error in (no error)=w1145, 9:20000 ("timeout ms (25000)")) -> (connection ID out=w1139:refnum<k5>, data out=w1136:string, error out=w1138:errorcluster)  [unwired: 1 in]
                n680 = TCP Close Connection(connection ID=w1139, error in (no error)=w1138) -> ()  [unwired: 1 in, 2 out]
                n681 = local write "data out"(w1136) -> ()
              }
              frame #3 {
                n682 = flat-sequence {
                  frame #0 {
                    n683 = TCP Open Connection(address="localhost", remote port or service name=u16 8089) -> (connection ID=w1152:refnum<k5>, error out=w1151:errorcluster)  [unwired: 3 in]
                    n684 = TCP Write(connection ID=w1152, data in="EXPS", error in (no error)=w1151) -> (connection ID out=w1157:refnum<k5>, error out=w1156:errorcluster)  [unwired: 1 in, 1 out]
                    n685 = TCP Read(connection ID=w1157, bytes to read=9, error in (no error)=w1156, 9:20000 ("timeout ms (25000)")) -> (connection ID out=w1150:refnum<k5>, data out=w1147:string, error out=w1149:errorcluster)  [unwired: 1 in]
                    n686 = local write "data out"(w1147) -> ()
                    n687 = TCP Close Connection(connection ID=w1150, error in (no error)=w1149) -> ()  [unwired: 1 in, 2 out]
                  }
                  frame #1 {
                    n688 = local read "Exposure ms"() -> (w1161:i32)
                    n689 = TCP Open Connection(address="localhost", remote port or service name=u16 8089) -> (connection ID=w1168:refnum<k5>, error out=w1169:errorcluster)  [unwired: 3 in]
                    n690 = Number To Decimal String(number=w1161) -> (decimal integer string=w1160:string)  [unwired: 1 in]
                    n691 = Format Into String(format string=" %4s", initial string=w1160, "") -> (resulting string=w1162:string)  [unwired: 1 in, 1 out]
                    n692 = TCP Write(connection ID=w1168, data in=w1162, error in (no error)=w1169) -> (connection ID out=w1163:refnum<k5>, error out=w1164:errorcluster)  [unwired: 1 in, 1 out]
                    n693 = TCP Read(connection ID=w1163, bytes to read=9, error in (no error)=w1164, 9:20000 ("timeout ms (25000)")) -> (connection ID out=w1170:refnum<k5>, data out=w1173:string, error out=w1171:errorcluster)  [unwired: 1 in]
                    n694 = local write "data out"(w1173) -> ()
                    n695 = TCP Close Connection(connection ID=w1170, error in (no error)=w1171) -> ()  [unwired: 1 in, 2 out]
                  }
                }
              }
              frame #4 {
                n696 = flat-sequence {
                  frame #0 {
                    n697 = TCP Open Connection(address="localhost", remote port or service name=u16 8089) -> (connection ID=w1180:refnum<k5>, error out=w1179:errorcluster)  [unwired: 3 in]
                    n698 = TCP Write(connection ID=w1180, data in="_DIR", error in (no error)=w1179) -> (connection ID out=w1185:refnum<k5>, error out=w1184:errorcluster)  [unwired: 1 in, 1 out]
                    n699 = TCP Read(connection ID=w1185, bytes to read=9, error in (no error)=w1184, 9:20000 ("timeout ms (25000)")) -> (connection ID out=w1178:refnum<k5>, data out=w1175:string, error out=w1177:errorcluster)  [unwired: 1 in]
                    n700 = local write "data out"(w1175) -> ()
                    n701 = TCP Close Connection(connection ID=w1178, error in (no error)=w1177) -> ()  [unwired: 1 in, 2 out]
                  }
                  frame #1 {
                    n702 = local read "fileName"() -> (w1191:path)
                    n703 = Path To String(path=w1191) -> (string=w1189:string)
                    n704 = TCP Open Connection(address="localhost", remote port or service name=u16 8089) -> (connection ID=w1197:refnum<k5>, error out=w1198:errorcluster)  [unwired: 3 in]
                    n705 = Format Into String(format string=" %1028s", initial string=w1189, "") -> (resulting string=w1190:string)  [unwired: 1 in, 1 out]
                    n706 = TCP Write(connection ID=w1197, data in=w1190, error in (no error)=w1198) -> (connection ID out=w1192:refnum<k5>, error out=w1193:errorcluster)  [unwired: 1 in, 1 out]
                    n707 = TCP Read(connection ID=w1192, bytes to read=9, error in (no error)=w1193, 9:20000 ("timeout ms (25000)")) -> (connection ID out=w1199:refnum<k5>, data out=w1202:string, error out=w1200:errorcluster)  [unwired: 1 in]
                    n708 = local write "data out"(w1202) -> ()
                    n709 = TCP Close Connection(connection ID=w1199, error in (no error)=w1200) -> ()  [unwired: 1 in, 2 out]
                  }
                }
              }
              frame #5 {
                # "LASER ON"
                n710 = TCP Open Connection(address="localhost", remote port or service name=u16 8089) -> (connection ID=w1209:refnum<k5>, error out=w1210:errorcluster)  [unwired: 3 in]
                n711 = TCP Write(connection ID=w1209, data in="L2ON" ("format string"), error in (no error)=w1210) -> (connection ID out=w1204:refnum<k5>, error out=w1205:errorcluster)  [unwired: 1 in, 1 out]
                n712 = TCP Read(connection ID=w1204, bytes to read=9, error in (no error)=w1205, 9:5000 ("timeout ms (25000)")) -> (connection ID out=w1211:refnum<k5>, data out=w1214:string, error out=w1212:errorcluster)  [unwired: 1 in]
                n713 = local write "data out"(w1214) -> ()
                n714 = TCP Close Connection(connection ID=w1211, error in (no error)=w1212) -> ()  [unwired: 1 in, 2 out]
              }
              frame #6 {
                # "Take a shot"
                n715 = TCP Open Connection(address="localhost", remote port or service name=u16 8089) -> (connection ID=w1220:refnum<k5>, error out=w1219:errorcluster)  [unwired: 3 in]
                n716 = TCP Write(connection ID=w1220, data in="IMGO", error in (no error)=w1219) -> (connection ID out=w1225:refnum<k5>, error out=w1224:errorcluster)  [unwired: 1 in, 1 out]
                n717 = TCP Read(connection ID=w1225, bytes to read=9, error in (no error)=w1224, 9:20000 ("timeout ms (25000)")) -> (connection ID out=w1218:refnum<k5>, data out=w1215:string, error out=w1217:errorcluster)  [unwired: 1 in]
                n718 = TCP Close Connection(connection ID=w1218, error in (no error)=w1217) -> ()  [unwired: 1 in, 2 out]
                n719 = local write "data out"(w1215) -> ()
              }
              frame #7 {
                # "LASER OFF"
                n720 = TCP Open Connection(address="localhost", remote port or service name=u16 8089) -> (connection ID=w1233:refnum<k5>, error out=w1234:errorcluster)  [unwired: 3 in]
                n721 = TCP Write(connection ID=w1233, data in="L2OF" ("format string"), error in (no error)=w1234) -> (connection ID out=w1228:refnum<k5>, error out=w1229:errorcluster)  [unwired: 1 in, 1 out]
                n722 = TCP Read(connection ID=w1228, bytes to read=9, error in (no error)=w1229, 9:5000 ("timeout ms (25000)")) -> (connection ID out=w1235:refnum<k5>, data out=w1238:string, error out=w1236:errorcluster)  [unwired: 1 in]
                n723 = local write "data out"(w1238) -> ()
                n724 = TCP Close Connection(connection ID=w1235, error in (no error)=w1236) -> ()  [unwired: 1 in, 2 out]
              }
              frame #8 {
                # "what is the length of the data?"
                n725 = TCP Open Connection(address="localhost", remote port or service name=u16 8089) -> (connection ID=w1245:refnum<k5>, error out=w1244:errorcluster)  [unwired: 3 in]
                n726 = TCP Write(connection ID=w1245, data in="GETL", error in (no error)=w1244) -> (connection ID out=w1250:refnum<k5>, error out=w1249:errorcluster)  [unwired: 1 in, 1 out]
                n727 = TCP Read(connection ID=w1250, bytes to read=20, error in (no error)=w1249, 9:5000 ("timeout ms (25000)")) -> (connection ID out=w1243:refnum<k5>, data out=w1240:string, error out=w1242:errorcluster)  [unwired: 1 in]
                n728 = Decimal String To Number(string=w1240) -> (number=w1239:i32)  [unwired: 2 in, 1 out]
                n729 = local write "data out"(w1240) -> ()
                n730 = TCP Close Connection(connection ID=w1243, error in (no error)=w1242) -> ()  [unwired: 1 in, 2 out]
                n731 = local write "length"(w1239) -> ()
              }
              frame #9 {
                # "get the data, plot the data"
                n732 = TCP Open Connection(address="localhost", remote port or service name=u16 8089) -> (connection ID=w1267:refnum<k5>, error out=w1268:errorcluster)  [unwired: 3 in]
                n733 = local read "length"() -> (w1269:i32)
                n734 = TCP Write(connection ID=w1267, data in="DATA", error in (no error)=w1268) -> (connection ID out=w1262:refnum<k5>, error out=w1263:errorcluster)  [unwired: 1 in, 1 out]
                n735 = TCP Read(connection ID=w1262, bytes to read=w1269, error in (no error)=w1263, 9:5000 ("timeout ms (25000)")) -> (data out=w1252:string)  [unwired: 1 in, 2 out]
                n736 = Spreadsheet String To Array(delimiter (Tab)=" ", format string="", spreadsheet string=w1252) -> (array=w1258:dbl[][])  [unwired: 1 in]
                n737 = local read "yo"() -> (w1253:i32)
                n738 = local read "xo"() -> (w1254:i32)
                n739 = To Long Integer(number=w1258) -> (32bit integer=w1257:i32[][])
                n740 = Reshape Array(w1257, w1253, w1254) -> (w1259:i32[][])
                n741 = To Long Integer(number=w1259) -> (32bit integer=w1260:i32[][])
                n742 = local write "Intensity OPT"(w1260) -> ()
              }
              frame #10 {
                # "Initialise the second laser, get the lambda"
                n743 = local write "lambda"(488.0 ("lambda")) -> ()
              }
              frame #11 {
                w1271 = "_" ("format string")
                # "Make the filename with the wavelength"
                n744 = local read "lambda"() -> (w1279:dbl)
                n745 = local read "Path"() -> (w1284:path)
                n746 = Increment(x=w1275) -> (x+1=w1277:i32)
                n747 = local read "File Prefix"() -> (w1282:string)
                n748 = Number To Decimal String(number=w1279) -> (decimal integer string=w1272:string)  [unwired: 1 in]
                n749 = Format Into String(format string="%03d", w1277) -> (resulting string=w1274:string)  [unwired: 2 in, 1 out]
                n750 = Path To String(path=w1284) -> (string=w1287:string)
                n751 = Format Date/Time String(time format string (%c)="%Y_%m_%d_%H_%M_%S") -> (date/time string=w1276:string)  [unwired: 2 in]
                n752 = local write "date/time string"(w1276) -> ()
                n753 = Concatenate Strings(w1287, "\\\\" ("format string"), w1282, w1271, w1274, "_2colour_" ("format string"), w1272, w1271) -> (w1286:string)
                n754 = String To Path(string=w1286) -> (path=w1285:path)
                n755 = call <vilib>:"Check if File or Folder Exists.vi"("path"=w1285) -> ("dup path"=w1280:path)  [unwired: 8 in, 2 out]
                n756 = case shown="True" TRUE {
                  tunnel: w1280 -> [w1289 w1291]
                  tunnel: [w1290 w1291] -> _
                  frame False {
                    n757 = Create Folder(path (use dialog)=w1289) -> (created path=w1290:path)  [unwired: 2 in, 2 out]
                  }
                  frame True {
                  }
                }
                n758 = local write "fileName"(w1280) -> ()
              }
              frame #12 {
                n759 = TCP Open Connection(address="localhost", remote port or service name=u16 8089) -> (connection ID=w1298:refnum<k5>, error out=w1297:errorcluster)  [unwired: 3 in]
                n760 = TCP Write(connection ID=w1298, data in="_OPT" ("format string"), error in (no error)=w1297) -> (connection ID out=w1303:refnum<k5>, error out=w1302:errorcluster)  [unwired: 1 in, 1 out]
                n761 = TCP Read(connection ID=w1303, bytes to read=9, error in (no error)=w1302, 9:20000 ("timeout ms (25000)")) -> (connection ID out=w1296:refnum<k5>, data out=w1293:string, error out=w1295:errorcluster)  [unwired: 1 in]
                n762 = TCP Close Connection(connection ID=w1296, error in (no error)=w1295) -> ()  [unwired: 1 in, 2 out]
                n763 = local write "data out"(w1293) -> ()
              }
              frame #13 {
                n764 = flat-sequence {
                  frame #0 {
                    n765 = TCP Open Connection(address="localhost", remote port or service name=u16 8089) -> (connection ID=w1309:refnum<k5>, error out=w1308:errorcluster)  [unwired: 3 in]
                    n766 = TCP Write(connection ID=w1309, data in="EXPS", error in (no error)=w1308) -> (connection ID out=w1314:refnum<k5>, error out=w1313:errorcluster)  [unwired: 1 in, 1 out]
                    n767 = TCP Read(connection ID=w1314, bytes to read=9, error in (no error)=w1313, 9:20000 ("timeout ms (25000)")) -> (connection ID out=w1307:refnum<k5>, data out=w1304:string, error out=w1306:errorcluster)  [unwired: 1 in]
                    n768 = local write "data out"(w1304) -> ()
                    n769 = TCP Close Connection(connection ID=w1307, error in (no error)=w1306) -> ()  [unwired: 1 in, 2 out]
                  }
                  frame #1 {
                    n770 = local read "Exposure ms"() -> (w1318:i32)
                    n771 = TCP Open Connection(address="localhost", remote port or service name=u16 8089) -> (connection ID=w1325:refnum<k5>, error out=w1326:errorcluster)  [unwired: 3 in]
                    n772 = Number To Decimal String(number=w1318) -> (decimal integer string=w1317:string)  [unwired: 1 in]
                    n773 = Format Into String(format string=" %4s", initial string=w1317, "") -> (resulting string=w1319:string)  [unwired: 1 in, 1 out]
                    n774 = TCP Write(connection ID=w1325, data in=w1319, error in (no error)=w1326) -> (connection ID out=w1320:refnum<k5>, error out=w1321:errorcluster)  [unwired: 1 in, 1 out]
                    n775 = TCP Read(connection ID=w1320, bytes to read=9, error in (no error)=w1321, 9:20000 ("timeout ms (25000)")) -> (connection ID out=w1327:refnum<k5>, data out=w1330:string, error out=w1328:errorcluster)  [unwired: 1 in]
                    n776 = local write "data out"(w1330) -> ()
                    n777 = TCP Close Connection(connection ID=w1327, error in (no error)=w1328) -> ()  [unwired: 1 in, 2 out]
                  }
                }
              }
              frame #14 {
                n778 = flat-sequence {
                  frame #0 {
                    n779 = TCP Open Connection(address="localhost", remote port or service name=u16 8089) -> (connection ID=w1337:refnum<k5>, error out=w1336:errorcluster)  [unwired: 3 in]
                    n780 = TCP Write(connection ID=w1337, data in="_DIR", error in (no error)=w1336) -> (connection ID out=w1342:refnum<k5>, error out=w1341:errorcluster)  [unwired: 1 in, 1 out]
                    n781 = TCP Read(connection ID=w1342, bytes to read=9, error in (no error)=w1341, 9:20000 ("timeout ms (25000)")) -> (connection ID out=w1335:refnum<k5>, data out=w1332:string, error out=w1334:errorcluster)  [unwired: 1 in]
                    n782 = local write "data out"(w1332) -> ()
                    n783 = TCP Close Connection(connection ID=w1335, error in (no error)=w1334) -> ()  [unwired: 1 in, 2 out]
                  }
                  frame #1 {
                    n784 = local read "fileName"() -> (w1348:path)
                    n785 = Path To String(path=w1348) -> (string=w1346:string)
                    n786 = TCP Open Connection(address="localhost", remote port or service name=u16 8089) -> (connection ID=w1354:refnum<k5>, error out=w1355:errorcluster)  [unwired: 3 in]
                    n787 = Format Into String(format string=" %1028s", initial string=w1346, "") -> (resulting string=w1347:string)  [unwired: 1 in, 1 out]
                    n788 = TCP Write(connection ID=w1354, data in=w1347, error in (no error)=w1355) -> (connection ID out=w1349:refnum<k5>, error out=w1350:errorcluster)  [unwired: 1 in, 1 out]
                    n789 = TCP Read(connection ID=w1349, bytes to read=9, error in (no error)=w1350, 9:20000 ("timeout ms (25000)")) -> (connection ID out=w1356:refnum<k5>, data out=w1359:string, error out=w1357:errorcluster)  [unwired: 1 in]
                    n790 = local write "data out"(w1359) -> ()
                    n791 = TCP Close Connection(connection ID=w1356, error in (no error)=w1357) -> ()  [unwired: 1 in, 2 out]
                  }
                }
              }
              frame #15 {
                # "LASER ON"
                n792 = TCP Open Connection(address="localhost", remote port or service name=u16 8089) -> (connection ID=w1366:refnum<k5>, error out=w1367:errorcluster)  [unwired: 3 in]
                n793 = TCP Write(connection ID=w1366, data in="L3ON" ("format string"), error in (no error)=w1367) -> (connection ID out=w1361:refnum<k5>, error out=w1362:errorcluster)  [unwired: 1 in, 1 out]
                n794 = TCP Read(connection ID=w1361, bytes to read=9, error in (no error)=w1362, 9:5000 ("timeout ms (25000)")) -> (connection ID out=w1368:refnum<k5>, data out=w1371:string, error out=w1369:errorcluster)  [unwired: 1 in]
                n795 = local write "data out"(w1371) -> ()
                n796 = TCP Close Connection(connection ID=w1368, error in (no error)=w1369) -> ()  [unwired: 1 in, 2 out]
              }
              frame #16 {
                # "Take a shot"
                n797 = TCP Open Connection(address="localhost", remote port or service name=u16 8089) -> (connection ID=w1377:refnum<k5>, error out=w1376:errorcluster)  [unwired: 3 in]
                n798 = TCP Write(connection ID=w1377, data in="IMGO", error in (no error)=w1376) -> (connection ID out=w1382:refnum<k5>, error out=w1381:errorcluster)  [unwired: 1 in, 1 out]
                n799 = TCP Read(connection ID=w1382, bytes to read=9, error in (no error)=w1381, 9:20000 ("timeout ms (25000)")) -> (connection ID out=w1375:refnum<k5>, data out=w1372:string, error out=w1374:errorcluster)  [unwired: 1 in]
                n800 = TCP Close Connection(connection ID=w1375, error in (no error)=w1374) -> ()  [unwired: 1 in, 2 out]
                n801 = local write "data out"(w1372) -> ()
              }
              frame #17 {
                # "LASER OFF"
                n802 = TCP Open Connection(address="localhost", remote port or service name=u16 8089) -> (connection ID=w1390:refnum<k5>, error out=w1391:errorcluster)  [unwired: 3 in]
                n803 = TCP Write(connection ID=w1390, data in="L3OF" ("format string"), error in (no error)=w1391) -> (connection ID out=w1385:refnum<k5>, error out=w1386:errorcluster)  [unwired: 1 in, 1 out]
                n804 = TCP Read(connection ID=w1385, bytes to read=9, error in (no error)=w1386, 9:5000 ("timeout ms (25000)")) -> (connection ID out=w1392:refnum<k5>, data out=w1395:string, error out=w1393:errorcluster)  [unwired: 1 in]
                n805 = local write "data out"(w1395) -> ()
                n806 = TCP Close Connection(connection ID=w1392, error in (no error)=w1393) -> ()  [unwired: 1 in, 2 out]
              }
              frame #18 {
                # "what is the length of the data?"
                n807 = TCP Open Connection(address="localhost", remote port or service name=u16 8089) -> (connection ID=w1402:refnum<k5>, error out=w1401:errorcluster)  [unwired: 3 in]
                n808 = TCP Write(connection ID=w1402, data in="GETL", error in (no error)=w1401) -> (connection ID out=w1407:refnum<k5>, error out=w1406:errorcluster)  [unwired: 1 in, 1 out]
                n809 = TCP Read(connection ID=w1407, bytes to read=20, error in (no error)=w1406, 9:5000 ("timeout ms (25000)")) -> (connection ID out=w1400:refnum<k5>, data out=w1397:string, error out=w1399:errorcluster)  [unwired: 1 in]
                n810 = Decimal String To Number(string=w1397) -> (number=w1396:i32)  [unwired: 2 in, 1 out]
                n811 = local write "data out"(w1397) -> ()
                n812 = TCP Close Connection(connection ID=w1400, error in (no error)=w1399) -> ()  [unwired: 1 in, 2 out]
                n813 = local write "length"(w1396) -> ()
              }
              frame #19 {
                # "get the data, plot the data"
                n814 = TCP Open Connection(address="localhost", remote port or service name=u16 8089) -> (connection ID=w1424:refnum<k5>, error out=w1425:errorcluster)  [unwired: 3 in]
                n815 = local read "length"() -> (w1426:i32)
                n816 = TCP Write(connection ID=w1424, data in="DATA", error in (no error)=w1425) -> (connection ID out=w1419:refnum<k5>, error out=w1420:errorcluster)  [unwired: 1 in, 1 out]
                n817 = TCP Read(connection ID=w1419, bytes to read=w1426, error in (no error)=w1420, 9:5000 ("timeout ms (25000)")) -> (data out=w1409:string)  [unwired: 1 in, 2 out]
                n818 = Spreadsheet String To Array(delimiter (Tab)=" ", format string="", spreadsheet string=w1409) -> (array=w1415:dbl[][])  [unwired: 1 in]
                n819 = local read "yo"() -> (w1410:i32)
                n820 = local read "xo"() -> (w1411:i32)
                n821 = To Long Integer(number=w1415) -> (32bit integer=w1414:i32[][])
                n822 = Reshape Array(w1414, w1410, w1411) -> (w1416:i32[][])
                n823 = To Long Integer(number=w1416) -> (32bit integer=w1417:i32[][])
                n824 = local write "Intensity OPT"(w1417) -> ()
              }
              frame #20 {
                n825 = property on="Two lambda old2" class="Bool (strict)"("Value"=FALSE ("Two lambda grab")) -> ()  [unwired: 2 in, 2 out]
                n826 = TCP Open Connection(address="localhost", remote port or service name=u16 8089) -> (connection ID=w1432:refnum<k5>, error out=w1431:errorcluster)  [unwired: 3 in]
                n827 = TCP Write(connection ID=w1432, data in="QUI_", error in (no error)=w1431) -> (connection ID out=w1437:refnum<k5>, error out=w1436:errorcluster)  [unwired: 1 in, 1 out]
                n828 = TCP Read(connection ID=w1437, bytes to read=9, error in (no error)=w1436, 9:5000 ("timeout ms (25000)")) -> (connection ID out=w1430:refnum<k5>, data out=w1428:string, error out=w1429:errorcluster)  [unwired: 1 in]
                n829 = local write "done"(w1428) -> ()
                n830 = TCP Close Connection(connection ID=w1430, error in (no error)=w1429) -> ()  [unwired: 1 in, 2 out]
              }
            }
          }
          event "Two lambda": Value Change {
            n831 = event-data() -> ()  [unwired: 1 in, 6 out]
            n832 = stacked-sequence {
              tunnel: w1440 -> [w1443 _ _ _ _ _ _]
              frame #0 {
                w1444 = "_" ("format string")
                # "Make the filename  with the wavelength"
                n833 = property on="Two lambda" class="Bool (strict)"("Value"=FALSE ("Two lambda")) -> ()  [unwired: 2 in, 2 out]
                n834 = local read "Path"() -> (w1453:path)
                n835 = Increment(x=w1443) -> (x+1=w1447:i32)
                n836 = local read "File Prefix"() -> (w1451:string)
                n837 = Format Into String(format string="%03d", w1447) -> (resulting string=w1446:string)  [unwired: 2 in, 1 out]
                n838 = Path To String(path=w1453) -> (string=w1456:string)
                n839 = Format Date/Time String(time format string (%c)="%Y_%m_%d_%H_%M_%S") -> (date/time string=w1457:string)  [unwired: 2 in]
                n840 = local write "date/time string"(w1457) -> ()
                n841 = Concatenate Strings(w1456, "\\\\" ("format string"), w1451, w1444, w1446, "_2colour_" ("format string"), "_" ("format string"), w1444) -> (w1455:string)
                n842 = String To Path(string=w1455) -> (path=w1454:path)
                n843 = call <vilib>:"Check if File or Folder Exists.vi"("path"=w1454) -> ("dup path"=w1449:path)  [unwired: 8 in, 2 out]
                n844 = case shown="True" TRUE {
                  tunnel: w1449 -> [w1459 w1461]
                  tunnel: [w1460 w1461] -> _
                  frame False {
                    n845 = Create Folder(path (use dialog)=w1459) -> (created path=w1460:path)  [unwired: 2 in, 2 out]
                  }
                  frame True {
                  }
                }
                n846 = local write "fileName"(w1449) -> ()
              }
              frame #1 {
                n847 = flat-sequence {
                  frame #0 {
                    n848 = TCP Open Connection(address="localhost", remote port or service name=u16 8089) -> (connection ID=w1467:refnum<k5>, error out=w1466:errorcluster)  [unwired: 3 in]
                    n849 = TCP Write(connection ID=w1467, data in="EXPS", error in (no error)=w1466) -> (connection ID out=w1472:refnum<k5>, error out=w1471:errorcluster)  [unwired: 1 in, 1 out]
                    n850 = TCP Read(connection ID=w1472, bytes to read=9, error in (no error)=w1471, 9:20000 ("timeout ms (25000)")) -> (connection ID out=w1465:refnum<k5>, data out=w1462:string, error out=w1464:errorcluster)  [unwired: 1 in]
                    n851 = local write "data out"(w1462) -> ()
                    n852 = TCP Close Connection(connection ID=w1465, error in (no error)=w1464) -> ()  [unwired: 1 in, 2 out]
                  }
                  frame #1 {
                    n853 = local read "Exposure ms"() -> (w1476:i32)
                    n854 = TCP Open Connection(address="localhost", remote port or service name=u16 8089) -> (connection ID=w1483:refnum<k5>, error out=w1484:errorcluster)  [unwired: 3 in]
                    n855 = Number To Decimal String(number=w1476) -> (decimal integer string=w1475:string)  [unwired: 1 in]
                    n856 = Format Into String(format string=" %4s", initial string=w1475, "") -> (resulting string=w1477:string)  [unwired: 1 in, 1 out]
                    n857 = TCP Write(connection ID=w1483, data in=w1477, error in (no error)=w1484) -> (connection ID out=w1478:refnum<k5>, error out=w1479:errorcluster)  [unwired: 1 in, 1 out]
                    n858 = TCP Read(connection ID=w1478, bytes to read=9, error in (no error)=w1479, 9:20000 ("timeout ms (25000)")) -> (connection ID out=w1485:refnum<k5>, data out=w1488:string, error out=w1486:errorcluster)  [unwired: 1 in]
                    n859 = local write "data out"(w1488) -> ()
                    n860 = TCP Close Connection(connection ID=w1485, error in (no error)=w1486) -> ()  [unwired: 1 in, 2 out]
                  }
                }
              }
              frame #2 {
                n861 = flat-sequence {
                  frame #0 {
                    n862 = TCP Open Connection(address="localhost", remote port or service name=u16 8089) -> (connection ID=w1495:refnum<k5>, error out=w1494:errorcluster)  [unwired: 3 in]
                    n863 = TCP Write(connection ID=w1495, data in="_DIR", error in (no error)=w1494) -> (connection ID out=w1500:refnum<k5>, error out=w1499:errorcluster)  [unwired: 1 in, 1 out]
                    n864 = TCP Read(connection ID=w1500, bytes to read=9, error in (no error)=w1499, 9:20000 ("timeout ms (25000)")) -> (connection ID out=w1493:refnum<k5>, data out=w1490:string, error out=w1492:errorcluster)  [unwired: 1 in]
                    n865 = local write "data out"(w1490) -> ()
                    n866 = TCP Close Connection(connection ID=w1493, error in (no error)=w1492) -> ()  [unwired: 1 in, 2 out]
                  }
                  frame #1 {
                    n867 = local read "fileName"() -> (w1506:path)
                    n868 = Path To String(path=w1506) -> (string=w1504:string)
                    n869 = TCP Open Connection(address="localhost", remote port or service name=u16 8089) -> (connection ID=w1512:refnum<k5>, error out=w1513:errorcluster)  [unwired: 3 in]
                    n870 = Format Into String(format string=" %1028s", initial string=w1504, "") -> (resulting string=w1505:string)  [unwired: 1 in, 1 out]
                    n871 = TCP Write(connection ID=w1512, data in=w1505, error in (no error)=w1513) -> (connection ID out=w1507:refnum<k5>, error out=w1508:errorcluster)  [unwired: 1 in, 1 out]
                    n872 = TCP Read(connection ID=w1507, bytes to read=9, error in (no error)=w1508, 9:20000 ("timeout ms (25000)")) -> (connection ID out=w1514:refnum<k5>, data out=w1517:string, error out=w1515:errorcluster)  [unwired: 1 in]
                    n873 = local write "data out"(w1517) -> ()
                    n874 = TCP Close Connection(connection ID=w1514, error in (no error)=w1515) -> ()  [unwired: 1 in, 2 out]
                  }
                }
              }
              frame #3 {
                n875 = local read "Colour 1"() -> (w1523:u16)
                n876 = local read "Colour 2"() -> (w1522:u16)
                n877 = case shown="2" w1522 {
                  tunnel: ["1" ("format string") "2" ("format string") "3" ("format string")] -> w1519
                  frame 0, Default {
                    n878 = local write "lambda"(561.0 ("lambda")) -> ()
                  }
                  frame 1 {
                    n879 = local write "lambda"(488.0 ("lambda")) -> ()
                  }
                  frame 2 {
                    n880 = local write "lambda"(404.0 ("lambda")) -> ()
                  }
                }
                n881 = case shown="0, Default" w1523 {
                  tunnel: ["1" ("format string") "2" ("format string") "3" ("format string")] -> w1520
                  frame 0, Default {
                    n882 = local write "lambda"(561.0 ("lambda")) -> ()
                  }
                  frame 1 {
                    n883 = local write "lambda"(488.0 ("lambda")) -> ()
                  }
                  frame 2 {
                    n884 = local write "lambda"(404.0 ("lambda")) -> ()
                  }
                }
                n885 = TCP Open Connection(address="localhost", remote port or service name=u16 8089) -> (connection ID=w1529:refnum<k5>, error out=w1528:errorcluster)  [unwired: 3 in]
                n886 = Concatenate Strings("TW" ("format string"), w1520, w1519) -> (w1518:string)
                n887 = TCP Write(connection ID=w1529, data in=w1518, error in (no error)=w1528) -> (connection ID out=w1534:refnum<k5>, error out=w1533:errorcluster)  [unwired: 1 in, 1 out]
                n888 = local write "commando"(w1518) -> ()
                n889 = TCP Read(connection ID=w1534, bytes to read=9, error in (no error)=w1533, 9:20000 ("timeout ms (25000)")) -> (connection ID out=w1527:refnum<k5>, data out=w1524:string, error out=w1526:errorcluster)  [unwired: 1 in]
                n890 = TCP Close Connection(connection ID=w1527, error in (no error)=w1526) -> ()  [unwired: 1 in, 2 out]
                n891 = local write "data out"(w1524) -> ()
              }
              frame #4 {
                # "what is the length of the data?"
                n892 = TCP Open Connection(address="localhost", remote port or service name=u16 8089) -> (connection ID=w1553:refnum<k5>, error out=w1552:errorcluster)  [unwired: 3 in]
                n893 = TCP Write(connection ID=w1553, data in="GETL", error in (no error)=w1552) -> (connection ID out=w1558:refnum<k5>, error out=w1557:errorcluster)  [unwired: 1 in, 1 out]
                n894 = TCP Read(connection ID=w1558, bytes to read=20, error in (no error)=w1557, 9:5000 ("timeout ms (25000)")) -> (connection ID out=w1551:refnum<k5>, data out=w1548:string, error out=w1550:errorcluster)  [unwired: 1 in]
                n895 = Decimal String To Number(string=w1548) -> (number=w1547:i32)  [unwired: 2 in, 1 out]
                n896 = local write "data out"(w1548) -> ()
                n897 = TCP Close Connection(connection ID=w1551, error in (no error)=w1550) -> ()  [unwired: 1 in, 2 out]
                n898 = local write "length"(w1547) -> ()
              }
              frame #5 {
                # "file path to the merged bmp"
                n899 = TCP Open Connection(address="localhost", remote port or service name=u16 8089) -> (connection ID=w1569:refnum<k5>, error out=w1570:errorcluster)  [unwired: 3 in]
                n900 = local read "length"() -> (w1571:i32)
                n901 = TCP Write(connection ID=w1569, data in="DATA", error in (no error)=w1570) -> (connection ID out=w1564:refnum<k5>, error out=w1565:errorcluster)  [unwired: 1 in, 1 out]
                n902 = TCP Read(connection ID=w1564, bytes to read=w1571, error in (no error)=w1565, 9:5000 ("timeout ms (25000)")) -> (data out=w1562:string)  [unwired: 1 in, 2 out]
                n903 = String To Path(string=w1562) -> (path=w1561:path)
                n904 = local write "pythonOut"(w1562) -> ()
                n905 = local write "fileNameMergedOPT"(w1561) -> ()
                n906 = property on="merged" class="Pict"("Visible"=TRUE) -> ()  [unwired: 2 in, 2 out]
              }
              frame #6 {
                n907 = local read "fileNameMergedOPT"() -> (w1574:path)
                n908 = call <vilib>:"Read BMP File.vi"("path to BMP file"=w1574) -> ("image data"=w1573:T5)  [unwired: 8 in, 2 out]
                n909 = call <vilib>:"Draw Flattened Pixmap.vi"("image data"=w1573) -> ("new picture"=w1572:picture)  [unwired: 8 in]
                n910 = local write "merged"(w1572) -> ()
              }
            }
          }
          event "show": Value Change {
            n911 = event-data() -> ()  [unwired: 1 in, 6 out]
            n912 = local read "show"() -> (w1575:bool)
            n913 = property on="merged" class="Pict"("Visible"=w1575) -> ()  [unwired: 2 in, 2 out]
          }
          event "Correlate": Value Change {
            n914 = event-data() -> ()  [unwired: 1 in, 6 out]
            n915 = property on="Correlate" class="Bool (strict)"("Value"=FALSE ("Correlate")) -> ()  [unwired: 2 in, 2 out]
            n916 = local read "fileNameMergedOPT"() -> (w1598:path)
            n917 = local read "fileNameFIBSEM"() -> (w1588:path)
            n918 = local read "Path"() -> (w1585:path)
            n919 = Increment(x=w1577) -> (x+1=w1581:i32)
            n920 = local read "File Prefix"() -> (w1583:string)
            n921 = Format Into String(format string="%03d", w1581) -> (resulting string=w1580:string)  [unwired: 2 in, 1 out]
            n922 = Path To String(path=w1585) -> (string=w1586:string)
            n923 = Path To String(path=w1598) -> (string=w1589:string)
            n924 = Path To String(path=w1588) -> (string=w1587:string)
            n925 = Concatenate Strings(w1586, "\\\\" ("format string"), w1583, "_" ("format string"), w1580, "_correlated.png" ("format string")) -> (w1576:string)
            n926 = Format Into String(format string=" \"%s\"  \"%s\" \"%s\" ", initial string="C:\\Users\\Admin\\MICROSCOPE\\DeMarcoLab\\correlateim\\dist\\main.exe" ("format string"), w1589, w1587, w1576) -> (resulting string=w1592:string, error out=w1595:errorcluster)  [unwired: 1 in]
            n927 = local write "commando"(w1592) -> ()
            n928 = call <vilib>:"System Exec.vi"("expected output size  (4096)"=u32 1, "run minimized? (F)"=TRUE, "wait until completion? (T)"=TRUE, "error in (no error)"=w1595, "command line"=w1592) -> ("standard output"=w1597:string)  [unwired: 3 in, 3 out]
            n929 = local write "pythonOut"(w1597) -> ()
          }
          event "Save OPT position": Value Change {
            n930 = event-data() -> ()  [unwired: 1 in, 6 out]
            n931 = TCP Open Connection(address="localhost", remote port or service name=u16 8089) -> (connection ID=w1606:refnum<k5>, error out=w1605:errorcluster)  [unwired: 3 in]
            n932 = TCP Write(connection ID=w1606, data in="POSO" ("format string"), error in (no error)=w1605) -> (connection ID out=w1611:refnum<k5>, error out=w1610:errorcluster)  [unwired: 1 in, 1 out]
            n933 = TCP Read(connection ID=w1611, bytes to read=9, error in (no error)=w1610, 9:20000 ("timeout ms (25000)")) -> (connection ID out=w1604:refnum<k5>, data out=w1601:string, error out=w1603:errorcluster)  [unwired: 1 in]
            n934 = TCP Close Connection(connection ID=w1604, error in (no error)=w1603) -> ()  [unwired: 1 in, 2 out]
            n935 = local write "data out"(w1601) -> ()
          }
          event "moveOPT": Value Change {
            n936 = event-data() -> ()  [unwired: 1 in, 6 out]
            n937 = property on="moveOPT" class="Bool (strict)"("Value"=FALSE ("moveOPT")) -> ()  [unwired: 2 in, 2 out]
            n938 = TCP Open Connection(address="localhost", remote port or service name=u16 8089) -> (connection ID=w1619:refnum<k5>, error out=w1618:errorcluster)  [unwired: 3 in]
            n939 = TCP Write(connection ID=w1619, data in="MOVO" ("format string"), error in (no error)=w1618) -> (connection ID out=w1624:refnum<k5>, error out=w1623:errorcluster)  [unwired: 1 in, 1 out]
            n940 = TCP Read(connection ID=w1624, bytes to read=9, error in (no error)=w1623, 9:20000 ("timeout ms (25000)")) -> (connection ID out=w1617:refnum<k5>, data out=w1614:string, error out=w1616:errorcluster)  [unwired: 1 in]
            n941 = TCP Close Connection(connection ID=w1617, error in (no error)=w1616) -> ()  [unwired: 1 in, 2 out]
            n942 = local write "data out"(w1614) -> ()
          }
          event "Save FIB position": Value Change {
            n943 = event-data() -> ()  [unwired: 1 in, 6 out]
            n944 = TCP Open Connection(address="localhost", remote port or service name=u16 8089) -> (connection ID=w1631:refnum<k5>, error out=w1630:errorcluster)  [unwired: 3 in]
            n945 = TCP Write(connection ID=w1631, data in="POSF" ("format string"), error in (no error)=w1630) -> (connection ID out=w1636:refnum<k5>, error out=w1635:errorcluster)  [unwired: 1 in, 1 out]
            n946 = TCP Read(connection ID=w1636, bytes to read=9, error in (no error)=w1635, 9:20000 ("timeout ms (25000)")) -> (connection ID out=w1629:refnum<k5>, data out=w1626:string, error out=w1628:errorcluster)  [unwired: 1 in]
            n947 = TCP Close Connection(connection ID=w1629, error in (no error)=w1628) -> ()  [unwired: 1 in, 2 out]
            n948 = local write "data out"(w1626) -> ()
          }
          event "moveFIB": Value Change {
            n949 = event-data() -> ()  [unwired: 1 in, 6 out]
            n950 = property on="moveFIB" class="Bool (strict)"("Value"=TRUE ("moveFIB")) -> ()  [unwired: 2 in, 2 out]
            n951 = TCP Open Connection(address="localhost", remote port or service name=u16 8089) -> (connection ID=w1644:refnum<k5>, error out=w1643:errorcluster)  [unwired: 3 in]
            n952 = TCP Write(connection ID=w1644, data in="MOVF" ("format string"), error in (no error)=w1643) -> (connection ID out=w1649:refnum<k5>, error out=w1648:errorcluster)  [unwired: 1 in, 1 out]
            n953 = TCP Read(connection ID=w1649, bytes to read=9, error in (no error)=w1648, 9:20000 ("timeout ms (25000)")) -> (connection ID out=w1642:refnum<k5>, data out=w1639:string, error out=w1641:errorcluster)  [unwired: 1 in]
            n954 = TCP Close Connection(connection ID=w1642, error in (no error)=w1641) -> ()  [unwired: 1 in, 2 out]
            n955 = local write "data out"(w1639) -> ()
          }
          event "Save LAMELLA position": Value Change {
            n956 = event-data() -> ()  [unwired: 1 in, 6 out]
            n957 = TCP Open Connection(address="localhost", remote port or service name=u16 8089) -> (connection ID=w1656:refnum<k5>, error out=w1655:errorcluster)  [unwired: 3 in]
            n958 = TCP Write(connection ID=w1656, data in="POSL" ("format string"), error in (no error)=w1655) -> (connection ID out=w1661:refnum<k5>, error out=w1660:errorcluster)  [unwired: 1 in, 1 out]
            n959 = TCP Read(connection ID=w1661, bytes to read=9, error in (no error)=w1660, 9:20000 ("timeout ms (25000)")) -> (connection ID out=w1654:refnum<k5>, data out=w1651:string, error out=w1653:errorcluster)  [unwired: 1 in]
            n960 = TCP Close Connection(connection ID=w1654, error in (no error)=w1653) -> ()  [unwired: 1 in, 2 out]
            n961 = local write "data out"(w1651) -> ()
          }
          event "moveLAMELLA": Value Change {
            n962 = event-data() -> ()  [unwired: 1 in, 6 out]
            n963 = property on="moveLAMELLA" class="Bool (strict)"("Value"=FALSE ("moveLAMELLA")) -> ()  [unwired: 2 in, 2 out]
            n964 = TCP Open Connection(address="localhost", remote port or service name=u16 8089) -> (connection ID=w1669:refnum<k5>, error out=w1668:errorcluster)  [unwired: 3 in]
            n965 = TCP Write(connection ID=w1669, data in="MOVL" ("format string"), error in (no error)=w1668) -> (connection ID out=w1674:refnum<k5>, error out=w1673:errorcluster)  [unwired: 1 in, 1 out]
            n966 = TCP Read(connection ID=w1674, bytes to read=9, error in (no error)=w1673, 9:20000 ("timeout ms (25000)")) -> (connection ID out=w1667:refnum<k5>, data out=w1664:string, error out=w1666:errorcluster)  [unwired: 1 in]
            n967 = TCP Close Connection(connection ID=w1667, error in (no error)=w1666) -> ()  [unwired: 1 in, 2 out]
            n968 = local write "data out"(w1664) -> ()
          }
          event "moveToOPT": Value Change {
            n969 = event-data() -> ()  [unwired: 1 in, 6 out]
            n970 = stacked-sequence {
              frame #0 {
                n971 = case shown="False" FALSE {
                  frame False {
                  }
                  frame True {
                    n972 = local read "Path to Autoscript"() -> (w1680:path)
                    n973 = local read "DX mm"() -> (w1677:dbl)
                    n974 = local read "DY mm"() -> (w1676:dbl)
                    n975 = Path To String(path=w1680) -> (string=w1684:string)
                    n976 = Format Into String(format string=" \"%s\" %f %f", initial string=w1684, "C:\\Users\\Admin\\MICROSCOPE\\pfib__Move_btw_FIB_OPT.py" ("Path to Function"), w1677, w1676) -> (resulting string=w1679:string, error out=w1683:errorcluster)  [unwired: 1 in]
                    n977 = local write "commando"(w1679) -> ()
                    n978 = call <vilib>:"System Exec.vi"("run minimized? (F)"=TRUE, "wait until completion? (T)"=TRUE, "error in (no error)"=w1683, "command line"=w1679) -> ("standard output"=w1686:string)  [unwired: 4 in, 3 out]
                    n979 = flat-sequence {
                      tunnel: w1686 -> [w1688]
                      frame #0 {
                        n980 = local write "pythonOut"(w1688) -> ()
                        n981 = local write "Ready"(TRUE ("Ready")) -> ()
                      }
                    }
                  }
                }
              }
              frame #1 {
                n982 = TCP Open Connection(address="localhost", remote port or service name=u16 8089) -> (connection ID=w1694:refnum<k5>, error out=w1693:errorcluster)  [unwired: 3 in]
                n983 = TCP Write(connection ID=w1694, data in="SHIF", error in (no error)=w1693) -> (connection ID out=w1699:refnum<k5>, error out=w1698:errorcluster)  [unwired: 1 in, 1 out]
                n984 = TCP Read(connection ID=w1699, bytes to read=9, error in (no error)=w1698, 9:20000 ("timeout ms (25000)")) -> (connection ID out=w1692:refnum<k5>, data out=w1689:string, error out=w1691:errorcluster)  [unwired: 1 in]
                n985 = local write "data out"(w1689) -> ()
                n986 = TCP Close Connection(connection ID=w1692, error in (no error)=w1691) -> ()  [unwired: 1 in, 2 out]
              }
              frame #2 {
                w1701 = FALSE ("moveToOPT")
                n987 = local read "DX mm"() -> (w1704:dbl)
                n988 = local read "DY mm"() -> (w1703:dbl)
                n989 = property on="moveToOPT" class="Bool (strict)"("Value"=w1701) -> ()  [unwired: 2 in, 2 out]
                n990 = local write "Ready"(w1701) -> ()
                n991 = Format Into String(format string="%.3f%s%.3f", w1704, " " ("format string"), w1703) -> (resulting string=w1706:string)  [unwired: 2 in, 1 out]
                n992 = Format Into String(format string=" %1028s", initial string=w1706, "") -> (resulting string=w1702:string)  [unwired: 1 in, 1 out]
                n993 = TCP Open Connection(address="localhost", remote port or service name=u16 8089) -> (connection ID=w1715:refnum<k5>, error out=w1716:errorcluster)  [unwired: 3 in]
                n994 = TCP Write(connection ID=w1715, data in=w1702, error in (no error)=w1716) -> (connection ID out=w1710:refnum<k5>, error out=w1711:errorcluster)  [unwired: 1 in, 1 out]
                n995 = TCP Read(connection ID=w1710, bytes to read=9, error in (no error)=w1711, 9:20000 ("timeout ms (25000)")) -> (connection ID out=w1717:refnum<k5>, data out=w1720:string, error out=w1718:errorcluster)  [unwired: 1 in]
                n996 = local write "data out"(w1720) -> ()
                n997 = TCP Close Connection(connection ID=w1717, error in (no error)=w1718) -> ()  [unwired: 1 in, 2 out]
              }
            }
          }
          event "moveToFIB": Value Change {
            n998 = event-data() -> ()  [unwired: 1 in, 6 out]
            n999 = stacked-sequence {
              frame #0 {
                n1000 = case shown="True" FALSE {
                  frame False {
                  }
                  frame True {
                    n1001 = local read "Path to Autoscript"() -> (w1730:path)
                    n1002 = local read "DX mm"() -> (w1728:dbl)
                    n1003 = local read "DY mm"() -> (w1724:dbl)
                    n1004 = Multiply(x=w1728, y=-1.0) -> (x*y=w1727:dbl)
                    n1005 = Multiply(x=w1724, y=-1.0) -> (x*y=w1722:dbl)
                    n1006 = Path To String(path=w1730) -> (string=w1734:string)
                    n1007 = Format Into String(format string=" \"%s\" %f %f", initial string=w1734, "C:\\Users\\Admin\\MICROSCOPE\\pfib__Move_btw_FIB_OPT.py" ("Path to Function"), w1727, w1722) -> (resulting string=w1726:string, error out=w1733:errorcluster)  [unwired: 1 in]
                    n1008 = local write "commando"(w1726) -> ()
                    n1009 = call <vilib>:"System Exec.vi"("run minimized? (F)"=TRUE, "wait until completion? (T)"=TRUE, "error in (no error)"=w1733, "command line"=w1726) -> ("standard output"=w1736:string)  [unwired: 4 in, 3 out]
                    n1010 = flat-sequence {
                      tunnel: w1736 -> [w1738]
                      frame #0 {
                        n1011 = local write "pythonOut"(w1738) -> ()
                        n1012 = local write "Ready"(TRUE ("Ready")) -> ()
                      }
                    }
                  }
                }
              }
              frame #1 {
                n1013 = TCP Open Connection(address="localhost", remote port or service name=u16 8089) -> (connection ID=w1744:refnum<k5>, error out=w1743:errorcluster)  [unwired: 3 in]
                n1014 = TCP Write(connection ID=w1744, data in="SHIF", error in (no error)=w1743) -> (connection ID out=w1749:refnum<k5>, error out=w1748:errorcluster)  [unwired: 1 in, 1 out]
                n1015 = TCP Read(connection ID=w1749, bytes to read=9, error in (no error)=w1748, 9:20000 ("timeout ms (25000)")) -> (connection ID out=w1742:refnum<k5>, data out=w1739:string, error out=w1741:errorcluster)  [unwired: 1 in]
                n1016 = local write "data out"(w1739) -> ()
                n1017 = TCP Close Connection(connection ID=w1742, error in (no error)=w1741) -> ()  [unwired: 1 in, 2 out]
              }
              frame #2 {
                w1757 = FALSE ("moveToFIB")
                n1018 = local read "DY mm"() -> (w1753:dbl)
                n1019 = local read "DX mm"() -> (w1755:dbl)
                n1020 = Multiply(x=w1755, y=-1.0) -> (x*y=w1752:dbl)
                n1021 = Multiply(x=w1753, y=-1.0) -> (x*y=w1751:dbl)
                n1022 = property on="moveToFIB" class="Bool (strict)"("Value"=w1757) -> ()  [unwired: 2 in, 2 out]
                n1023 = local write "Ready"(w1757) -> ()
                n1024 = Format Into String(format string="%.3f%s%.3f", w1752, " " ("format string"), w1751) -> (resulting string=w1760:string)  [unwired: 2 in, 1 out]
                n1025 = Format Into String(format string=" %1028s", initial string=w1760, "") -> (resulting string=w1758:string)  [unwired: 1 in, 1 out]
                n1026 = TCP Open Connection(address="localhost", remote port or service name=u16 8089) -> (connection ID=w1769:refnum<k5>, error out=w1770:errorcluster)  [unwired: 3 in]
                n1027 = TCP Write(connection ID=w1769, data in=w1758, error in (no error)=w1770) -> (connection ID out=w1764:refnum<k5>, error out=w1765:errorcluster)  [unwired: 1 in, 1 out]
                n1028 = TCP Read(connection ID=w1764, bytes to read=9, error in (no error)=w1765, 9:20000 ("timeout ms (25000)")) -> (connection ID out=w1771:refnum<k5>, data out=w1774:string, error out=w1772:errorcluster)  [unwired: 1 in]
                n1029 = local write "data out"(w1774) -> ()
                n1030 = TCP Close Connection(connection ID=w1771, error in (no error)=w1772) -> ()  [unwired: 1 in, 2 out]
              }
            }
          }
          event "HOME": Value Change {
            w1781 = u32 0 ("channelIndex")
            n1031 = event-data() -> ()  [unwired: 1 in, 6 out]
            n1032 = call "sub - INITIALIZE linear.vi"("Zero?"=TRUE, "error in (no error)"=w1779, "channelIndex"=w1781, "systemIndex"=w1778) -> ("error out"=w1780:errorcluster, "systemIndexOut"=w1782:u32)  [unwired: 1 out]
            n1033 = property on="HOME" class="Bool (strict)"("Value"=FALSE ("HOME")) -> ()  [unwired: 2 in, 2 out]
            n1034 = call <vilib>:"SA_GetPosition_S.vi"("channelIndex"=w1781, "systemIndex"=w1782, "error in (no error)"=w1780) -> ("position"=w1776:i32)  [unwired: 7 in, 1 out]
            n1035 = property on="z um" class="DigNum (strict)"("Value"=w1776) -> ()  [unwired: 2 in, 2 out]
            n1036 = global write "Globals.vi" "X"(w1776) -> ()
          }
        }
        n1037 = global read "Globals.vi" "moving"() -> (→"moving":bool)
      }
    }
  }
  n1038 = while {
    stop <- w1784 stop-if-true
    n1039 = event shown="[1] \"ON/OFF\": Value Change" {
      selector: _ -> [_ _ _ _ _ _]
      dyn-events: _ -> [_ _ _ _ _ _]
      timeout: _ -> [_ _ _ _ _ _]
      tunnel: [_ _ _ _ _ w1856] -> w1784
      event Timeout {
        n1040 = event-data() -> ()  [unwired: 1 in, 3 out]
      }
      event "ON/OFF": Value Change {
        n1041 = event-data() -> ()  [unwired: 1 in, 6 out]
        n1042 = local read "Colour"() -> (w1789:u16)
        n1043 = local read "ON/OFF"() -> (w1788:bool)
        n1044 = case shown="0, Default" w1789 {
          tunnel: ["L2" ("format string") "L3" ("format string") "L4" ("format string")] -> w1787
          frame 0, Default {
            n1045 = local write "lambda"(561.0 ("lambda")) -> ()
          }
          frame 1 {
            n1046 = local write "lambda"(488.0 ("lambda")) -> ()
          }
          frame 2 {
            n1047 = local write "lambda"(404.0 ("lambda")) -> ()
          }
        }
        n1048 = case shown="True" w1788 {
          tunnel: ["OF" ("format string") "ON" ("format string")] -> w1786
          frame False {
          }
          frame True {
          }
        }
        n1049 = Format Into String(initial string=w1787, w1786) -> (resulting string=w1785:string)  [unwired: 2 in, 1 out]
        n1050 = TCP Open Connection(address="localhost", remote port or service name=u16 8089) -> (connection ID=w1795:refnum<k5>, error out=w1794:errorcluster)  [unwired: 3 in]
        n1051 = TCP Write(connection ID=w1795, data in=w1785, error in (no error)=w1794) -> (connection ID out=w1800:refnum<k5>, error out=w1799:errorcluster)  [unwired: 1 in, 1 out]
        n1052 = TCP Read(connection ID=w1800, bytes to read=9, error in (no error)=w1799, 9:5000 ("timeout ms (25000)")) -> (connection ID out=w1793:refnum<k5>, data out=w1790:string, error out=w1792:errorcluster)  [unwired: 1 in]
        n1053 = local write "data out"(w1790) -> ()
        n1054 = TCP Close Connection(connection ID=w1793, error in (no error)=w1792) -> ()  [unwired: 1 in, 2 out]
      }
      event "Power %": Mouse Down {
        n1055 = event-data() -> ()  [unwired: 1 in, 8 out]
        n1056 = local write "LASmouseDOWN"(TRUE ("L1mouse")) -> ()
      }
      event "Power %": Mouse Up {
        n1057 = event-data() -> ()  [unwired: 1 in, 8 out]
        n1058 = local read "LASmouseDOWN"() -> (w1810:bool)
        n1059 = case shown="True" w1810 {
          frame False {
          }
          frame True {
            n1060 = stacked-sequence {
              frame #0 {
                n1061 = local write "LASmouseDOWN"(FALSE ("LASmouse")) -> ()
                n1062 = local read "Colour"() -> (w1812:u16)
                n1063 = case shown="0, Default" w1812 {
                  tunnel: ["L2PW" ("format string") "L3PW" ("format string") "L4PW" ("format string")] -> w1811
                  frame 0, Default {
                  }
                  frame 1 {
                  }
                  frame 2 {
                  }
                }
                n1064 = TCP Open Connection(address="localhost", remote port or service name=u16 8089) -> (connection ID=w1818:refnum<k5>, error out=w1819:errorcluster)  [unwired: 3 in]
                n1065 = TCP Write(connection ID=w1818, data in=w1811, error in (no error)=w1819) -> (connection ID out=w1813:refnum<k5>, error out=w1814:errorcluster)  [unwired: 1 in, 1 out]
                n1066 = TCP Read(connection ID=w1813, bytes to read=9, error in (no error)=w1814, 9:20000 ("timeout ms (25000)")) -> (connection ID out=w1820:refnum<k5>, data out=w1823:string, error out=w1821:errorcluster)  [unwired: 1 in]
                n1067 = local write "data out"(w1823) -> ()
                n1068 = TCP Close Connection(connection ID=w1820, error in (no error)=w1821) -> ()  [unwired: 1 in, 2 out]
              }
              frame #1 {
                n1069 = local read "Power %"() -> (w1830:dbl)
                n1070 = TCP Open Connection(address="localhost", remote port or service name=u16 8089) -> (connection ID=w1837:refnum<k5>, error out=w1838:errorcluster)  [unwired: 3 in]
                n1071 = Number To Decimal String(number=w1830) -> (decimal integer string=w1829:string)  [unwired: 1 in]
                n1072 = Format Into String(format string=" %1028s", initial string=w1829, "") -> (resulting string=w1831:string)  [unwired: 1 in, 1 out]
                n1073 = TCP Write(connection ID=w1837, data in=w1831, error in (no error)=w1838) -> (connection ID out=w1832:refnum<k5>, error out=w1833:errorcluster)  [unwired: 1 in, 1 out]
                n1074 = TCP Read(connection ID=w1832, bytes to read=9, error in (no error)=w1833, 9:20000 ("timeout ms (25000)")) -> (connection ID out=w1839:refnum<k5>, data out=w1842:string, error out=w1840:errorcluster)  [unwired: 1 in]
                n1075 = local write "data out"(w1842) -> ()
                n1076 = TCP Close Connection(connection ID=w1839, error in (no error)=w1840) -> ()  [unwired: 1 in, 2 out]
              }
            }
          }
        }
      }
      event "Quit TCP": Value Change {
        n1077 = event-data() -> ()  [unwired: 1 in, 6 out]
        n1078 = TCP Open Connection(address="localhost", remote port or service name=u16 8089) -> (connection ID=w1848:refnum<k5>, error out=w1847:errorcluster)  [unwired: 3 in]
        n1079 = TCP Write(connection ID=w1848, data in="QUIT", error in (no error)=w1847) -> (connection ID out=w1853:refnum<k5>, error out=w1852:errorcluster)  [unwired: 1 in, 1 out]
        n1080 = TCP Read(connection ID=w1853, bytes to read=9, error in (no error)=w1852, 9:5000 ("timeout ms (25000)")) -> (connection ID out=w1846:refnum<k5>, data out=w1844:string, error out=w1845:errorcluster)  [unwired: 1 in]
        n1081 = local write "done"(w1844) -> ()
        n1082 = TCP Close Connection(connection ID=w1846, error in (no error)=w1845) -> ()  [unwired: 1 in, 2 out]
      }
      event "STOP": Value Change {
        n1083 = event-data() -> ("NewVal"=w1856:bool)  [unwired: 1 in, 5 out]
      }
    }
  }
  n1084 = while {
    stop <- w1857 stop-if-true
    n1085 = event shown="[2] \"Power L1 %\": Mouse Up" {
      selector: _ -> [_ _ _ _ _]
      dyn-events: _ -> [_ _ _ _ _]
      timeout: _ -> [_ _ _ _ _]
      tunnel: [w1862 _ _ _ _] -> w1857
      event "STOP": Value Change {
        w1858 = FALSE ("L1")
        n1086 = event-data() -> ("NewVal"=w1862:bool)  [unwired: 1 in, 5 out]
        n1087 = local write "L1"(w1858) -> ()
        n1088 = local read "error Obis"() -> (w1860:errorcluster)
        n1089 = local read "Laser"() -> (w1861:refnum<visa-resource-name>)
        n1090 = local write "Obis"(w1858) -> ()
        n1091 = VISA Close(VISA resource name=w1861, error in (no error)=w1860) -> (error out=w1859:errorcluster)
        n1092 = local write "error Obis"(w1859) -> ()
      }
      event "Power L1 %": Mouse Down {
        n1093 = event-data() -> ()  [unwired: 1 in, 8 out]
        n1094 = local write "LASmouseDOWN"(TRUE ("L1mouse")) -> ()
      }
      event "Power L1 %": Mouse Up {
        n1095 = event-data() -> ()  [unwired: 1 in, 8 out]
        n1096 = local read "LASmouseDOWN"() -> (w1864:bool)
        n1097 = case shown="True" w1864 {
          frame False {
          }
          frame True {
            n1098 = local read "Power1max"() -> (w1875:dbl)
            n1099 = local read "Power L1 %"() -> (w1872:i32)
            n1100 = local write "LASmouseDOWN"(FALSE ("LASmouse")) -> ()
            n1101 = Divide(x=w1875, y=110.0) -> (x/y=w1873:dbl)
            n1102 = local read "baud rate Obis"() -> (w1866:u32)
            n1103 = Multiply(x=w1873, y=w1872) -> (x*y=w1871:dbl)
            n1104 = local read "error Obis"() -> (w1870:errorcluster)
            n1105 = local read "Laser"() -> (w1876:refnum<visa-resource-name>)
            n1106 = call "sub - Laser Set Power Level.vi"("VISA resource name"=w1876, "baud rate (9600)"=w1866, "POWER"=w1871, "error in (no error)"=w1870) -> ("reference out"=w1867:refnum<visa-resource-name>, "message"=w1869:string, "Power"=w1868:dbl, "error out"=w1865:errorcluster)  [unwired: 1 out]
            n1107 = local write "Message Obis"(w1869) -> ()
            n1108 = local write "Obis out"(w1867) -> ()
            n1109 = local write "error Obis"(w1865) -> ()
            n1110 = local write "Power"(w1868) -> ()
          }
        }
      }
      event "ON/OFF 3": Value Change {
        n1111 = event-data() -> ()  [unwired: 1 in, 6 out]
        n1112 = local read "baud rate Obis"() -> (w1879:u32)
        n1113 = local read "error Obis"() -> (w1887:errorcluster)
        n1114 = local read "ON/OFF 3"() -> (w1881:bool)
        n1115 = local read "Laser"() -> (w1888:refnum<visa-resource-name>)
        n1116 = call "sub - Laser ON or OFF.vi"("error in (no error)"=w1887, "ON/OFF"=w1881, "baud rate (9600)"=w1879, "VISA resource name"=w1888) -> ("error out"=w1878:errorcluster, "message"=w1884:string, "reference out"=w1880:refnum<visa-resource-name>)  [unwired: 1 out]
        n1117 = String Subset(string=w1884, length (rest)=2 ("length (rest)")) -> (substring=w1882:string)  [unwired: 1 in]
        n1118 = Equal?(x=w1882, y="OK") -> (x = y?=w1885:bool)
        n1119 = local write "Message Obis"(w1884) -> ()
        n1120 = local write "error Obis"(w1878) -> ()
        n1121 = case shown="True" w1885 {
          tunnel: w1880 -> [_ w1893]
          tunnel: w1878 -> [_ w1896]
          tunnel: w1879 -> [_ w1891]
          frame False {
            n1122 = local write "Obis"(FALSE ("Obis")) -> ()
          }
          frame True {
            n1123 = call "sub - Laser Get Status ON or OFF.vi"("VISA resource name"=w1893, "baud rate (9600)"=w1891, "error in (no error)"=w1896) -> ("reference out"=w1892:refnum<visa-resource-name>, "ON/OFF"=w1895:bool, "message"=w1894:string, "error out"=w1890:errorcluster)  [unwired: 1 out]
            n1124 = local write "Message Obis"(w1894) -> ()
            n1125 = local write "error Obis"(w1890) -> ()
            n1126 = local write "Obis out"(w1892) -> ()
            n1127 = local write "L1"(w1895) -> ()
          }
        }
      }
      event "Laser": Value Change {
        n1128 = event-data() -> ()  [unwired: 1 in, 6 out]
        n1129 = local read "baud rate Obis"() -> (w1909:u32)
        n1130 = local read "Laser"() -> (w1903:refnum<visa-resource-name>)
        n1131 = call "sub - Laser Get WaveLength.vi"("VISA resource name"=w1903, "baud rate (9600)"=w1909) -> ("reference out"=w1920:refnum<visa-resource-name>, "wavelength"=w1917:dbl, "error out"=w1905:errorcluster, "message"=w1904:string)  [unwired: 1 in, 1 out]
        n1132 = call "sub - Laser Get Power Limits.vi"("VISA resource name"=w1920, "baud rate (9600)"=w1909, "error in (no error)"=w1905) -> ("powerNominal"=w1911:dbl, "powerMin"=w1906:dbl, "powerMax"=w1907:dbl, "error out"=w1908:errorcluster)  [unwired: 1 out]
        n1133 = local write "lambda"(w1917) -> ()
        n1134 = call "sub - Laser Get Power.vi"("VISA resource name"=w1920, "baud rate (9600)"=w1909, "error in (no error)"=w1908) -> ("reference out"=w1899:refnum<visa-resource-name>, "Power"=w1910:dbl, "error out"=w1898:errorcluster)  [unwired: 2 out]
        n1135 = call "sub - Laser Get Status ON or OFF.vi"("VISA resource name"=w1899, "error in (no error)"=w1898) -> ("reference out"=w1901:refnum<visa-resource-name>, "ON/OFF"=w1897:bool, "message"=w1902:string, "error out"=w1900:errorcluster)  [unwired: 1 in, 1 out]
        n1136 = Format Into String(format string="%d", w1917) -> (resulting string=w1921:string)  [unwired: 2 in, 1 out]
        n1137 = local write "Power1max"(w1907) -> ()
        n1138 = local write "PowerNom1"(w1911) -> ()
        n1139 = local write "Power1min"(w1906) -> ()
        n1140 = local write "Message Obis"(w1902) -> ()
        n1141 = local write "error Obis"(w1900) -> ()
        n1142 = local write "Obis out"(w1901) -> ()
        n1143 = local write "L1"(w1897) -> ()
        n1144 = local write "Message Obis"(w1904) -> ()
        n1145 = local write "Power"(w1910) -> ()
        n1146 = Concatenate Strings("wav" ("string"), w1921) -> (w1919:string)
        n1147 = property on="ON/OFF 3" class="Bool (strict)"("Value"=w1897) -> ()  [unwired: 2 in, 2 out]
        n1148 = local write "wav 1"(w1919) -> ()
        n1149 = Divide(x=w1910, y=w1911) -> (x/y=w1912:dbl)
        n1150 = Multiply(x=w1912, y=100.0) -> (x*y=w1915:dbl)
        n1151 = To Long Integer(number=w1915) -> (32bit integer=w1914:i32)
        n1152 = local write "Power L1 %"(w1914) -> ()
      }
    }
  }
  n1153 = call <vilib>:"SA_CloseSystem.vi"("systemIndex"=w24, "error in (no error)"=w23) -> ("error out"=w25:errorcluster)  [unwired: 9 in]
  n1154 = local write "error stage"(w25) -> ()
  "L1" <- FALSE ("L1")
  "Obis" <- FALSE ("Obis")
  "LASmouseDOWN" <- FALSE ("Mouse Down")
  "Ready" <- FALSE ("Ready")
